vi "信号光谱9-Au-卍  -MoO3.vi"() -> ()   [LabVIEW 2018]
uses:
  <vilib>/Utility/NIReport.llb/Report Type.ctl
  <vilib>/Utility/file.llb/Write Delimited Spreadsheet (DBL).vi
  <vilib>/Instr/_visa.llb/VISA Configure Serial Port (Instr).vi
  <vilib>/addons/_office/excel.llb/Excel Get Data ([str]).vi
  <vilib>/Utility/NIReport.llb/NI_report.lvclass
  <vilib>/Analysis/NI_AALBase.lvlib
  <vilib>/ptbypt/NI_PtbyPt.lvlib
  <vilib>/Utility/NIReport.llb/NI_ReportGenerationCore.lvlib
  <vilib>/addons/_office/NI_ReportGenerationToolkit.lvlib
  <vilib>/Utility/NIReport.llb/Excel/NI_Excel.lvclass
panel:
  in  "CW":i32=1
  out "temp":i32
  in  "num":i32=2
  in  "角度判断下限":dbl=1.0 format="%#_13g"
  in  "角度判断上限":dbl=4.0 format="%#_13g"
  out "原始峰值":dbl
  out "拟合峰值":dbl
  in  "角度倍乘系数":dbl=1.5
  out "结果展示":dbl[][](array[numeric])=[[37.33100777239877, 2672.955043835526, 29.54153292599307, 222755.0, 50.0], [37.36593979472361, 2672.656498058864, 30.113284142729572, 222833.0, 50.0], [38.96986225690859, 2673.3337152325566, 33.38805102415213, 222910.0, 75.0], [37.39946104045098, 2676.4005085744548, 31.215565446104666, 222948.0, 47.0], [35.862209164247574, 2671.7826876859012, 30.355582265151796, 223028.0, 47.0]]
  out "Δw2>C":bool=TRUE
  out "Δw1>C":bool=TRUE
  out "θi":dbl
  in  "w0":dbl format="%#_13g"
  in  "C=w-w0":dbl=1800.0 format="%#_13g"
  in  "上升下降沿/s":dbl format="%.2p"
  in  "延时/s":dbl format="%.2p"
  in  "占空比/%":dbl=3.0 format="%.2p"
  in  "高电平/V":dbl=4.0 format="%.2p"
  in  "频率/Hz":dbl=6000.0 format="%.3p"
  in  "低电平/V":dbl min=0.0 max=5.0 format="%.2p"
  in  "Enable":bool
  in  "上升下降沿":i32(ring)=1 items=["上升沿", "下降沿"]
  in  "输出信号波形":u16(ring) items=["Pulse"]
  out "Output":bool
  in  "VISA 信号发生器":refnum<visa-resource-name>="USB0::0x1AB1::0x0641::DG4E192200870::INSTR"
  out "Output 2":bool
  in  "Enable 2":bool
  in  "上升下降沿/s 2":dbl format="%.2p"
  in  "延时/s 2":dbl format="%.2p"
  in  "占空比/% 2":dbl=3.0 format="%.2p"
  in  "高电平/V 2":dbl=0.002 format="%.2p"
  in  "频率/Hz 2":dbl=6000.0 format="%.3p"
  in  "低电平/V 2":dbl min=0.0 max=5.0 format="%.2p"
  in  "上升下降沿 2":i32(ring)=1 items=["上升沿", "下降沿"]
  in  "输出信号波形 2":u16(ring) items=["Pulse"]
  in  "终止测量":bool
  in  "测量次数":i32=1
  out "best fit":cluster{"Y":dbl[], "Y":dbl[]}[](graph)
  in  "拟合终点":i32=850
  in  "拟合起点":i32=200
  out "angle":dbl
  out "图片地址":string
  in  "开光时间/ms":u32=50
  out "最终存储路径 2":path
  out "照明光error out":errorcluster
  in  "照明光":bool
  in  "stop bits (10: 1 bit)":u16(ring)=10 items=["1.0"=10, "1.5"=15, "2.0"=20]
  in  "parity (0:none)":enum16{"None", "Odd", "Even", "Mark", "Space"}(ring)
  in  "data bits (8)":u16=8 min=5 max=8 step=1
  in  "baud rate":u32=9600 caption="baud rate (115200)" min=9600 max=115200
  in  "照明光VISA":refnum<visa-resource-name>="COM13"
  out "正在测量":bool
  in  "滤波阈值":dbl=3000.0 format="%#_13g"
  out "范围内？":bool[](array[boolean])
  out "w":dbl
  out "xc":dbl
  out "拟合参数":dbl[](array[numeric])
  out "最终存储路径":path
  in  "停止程序":bool
  out "configure error out":errorcluster
  in  "设置参数":bool
  out "output control error  4":errorcluster
  in  "低电平持续输出":bool
  out "output control error  5":errorcluster
  out "output control error":errorcluster
  in  "开始测量":bool
  in  "channel输出口":i32(ring) items=["Channel 1", "Channel 2"]
  out "output control error":errorcluster
  out "Spectrum":cluster{"Y":dbl[], "Y":dbl[]}[](graph)
  out "波长范围":dbl[](array[numeric])
  in  "?":enum32{"IHR 550", "CCD"}(tab)
  in  "Move To\nTarget Positions":bool
  out "Current UniqueID":string="Mono4"
  in  "Mono ID":string(combo)="Mono1"
  in  "Connect":bool
  out "Initialized JY":bool=TRUE
  in  "Force\nInitialization":bool
  in  "Target Grating":string(combo)="2"
  out "Current Description":string="1" caption="Description"
  out "Grating Index":i32=1
  out "Current Grating":dbl=1200.0
  out "Units":string="nm"
  out "Current WL":dbl=897.9988
  out "Exit Mirror\nPosition":i32(ring)=2 items=["EntranceMirror", "ExitMirror", "Front", "Side"]
  out "Entrance Mirror\nPosition":i32(ring)=2 items=["EntranceMirror", "ExitMirror", "Front", "Side"]
  out "Units 2":string="mm"
  out "Front Entrance":dbl
  in  "Target WL":dbl=516.0
  in  "Exit Mirror":u16(ring)=3 caption="Target Position Exit Mirror" items=["Front"=2, "Side"=3]
  in  "Entrance Mirror":u16(ring)=2 caption="Target Position\nEntrance Mirror" items=["Front"=2, "Side"=3]
  in  "Target\nFront Entrance":dbl=2.0
  in  "Commande tab":T1(tab)
  in  "Area Number to Display":i32
  in  "Reformat":bool
  in  "GAIN":u16(ring)=2 caption="Device Name" items=["High Light", "Best Dynamic Range", "High Sensitivity"]
  in  "ADC":u16(ring) caption="Device Name" items=["20 kHz       ", " 1 MHz       ", " 1 MHz Ultra "]
  in  "Number of Areas :":u16=1 min=1 step=1
  in  "Integration time (ms) :":i16=5000
  out "Uniques ID":u16(ring) items=["CCD1", "CCD2"]
  in  "Device Name":u16(ring) items=["Synapse CCD (Lateral)", "Synapse_IGA (Axial)"]
  in  "Signal type :":enum16{"TTL Rising Edge", "TTL Falling Edge"}(ring)=enum."TTL Falling Edge"
  in  "Trigger Type :":u16(ring) items=["On Start"=1, "Per Acquisition"=2]
  in  "trigSigTypeString":string
  in  "trigEventString":string
  in  "Enable InputTriggers :":bool
  in  "Number of Cleans":i32=1
  in  "MultiAcqShutterMode":i32(ring)=3 items=["Open For All Spectra"=1, "Open for Each Spectrum"=3]
  in  "Accumulations:":u16=10 min=1 step=1
  in  "Multi Accumulation mode:":bool
  out "Y Pixels:":i32=256
  out "DataSize":i32=1024
  out "X Pixels:":i32=1024
  out "Firmware\nVersion":string="V1.20 CCD_4000"
  out "initialized ?":bool=TRUE
  in  "Continuous":bool
  in  "CCD Busy":bool
  out "indicator":string="Ready !"
  in  "initialize":bool
  in  "ShutterOpen":bool=TRUE caption="Shutter enable"
  in  "Acquire":bool
  in  "Temperature":bool
  in  "Setup":bool
  out "Acq Time(ms)":u32=3401
  in  "Save Backlight":bool
  in  "cut backlight":bool
  out "backlight":bool=TRUE
  in  "是否拟合":bool
  in  "是否保存":bool
  in  "Close":bool=TRUE
  out "JYCCDLib.IJYCCDReqd":refnum<k7>
  out "areas :":i32[][](array[numeric])=[[1], [1], [1], [1024], [256], [1], [256]]
  in  "Constante de condition\n(Voir l'aide contextuelle)":bool
  out "temp graph":dbl(graph)=-134.538067
  out "ADC Number":i32[](array[numeric])=[0, 1, 2, 3, 4]
  out "Gain Number":i32[](array[numeric])=[10, 11, 12, 13, 8, 2]
  out "trigAddress":i32
  out "Data":i32[][](graph)
  out "error out":errorcluster
  out "Gratings":dbl[](array[numeric])=[1200.0, 300.0]
  out "Backlight":i32[][](graph)
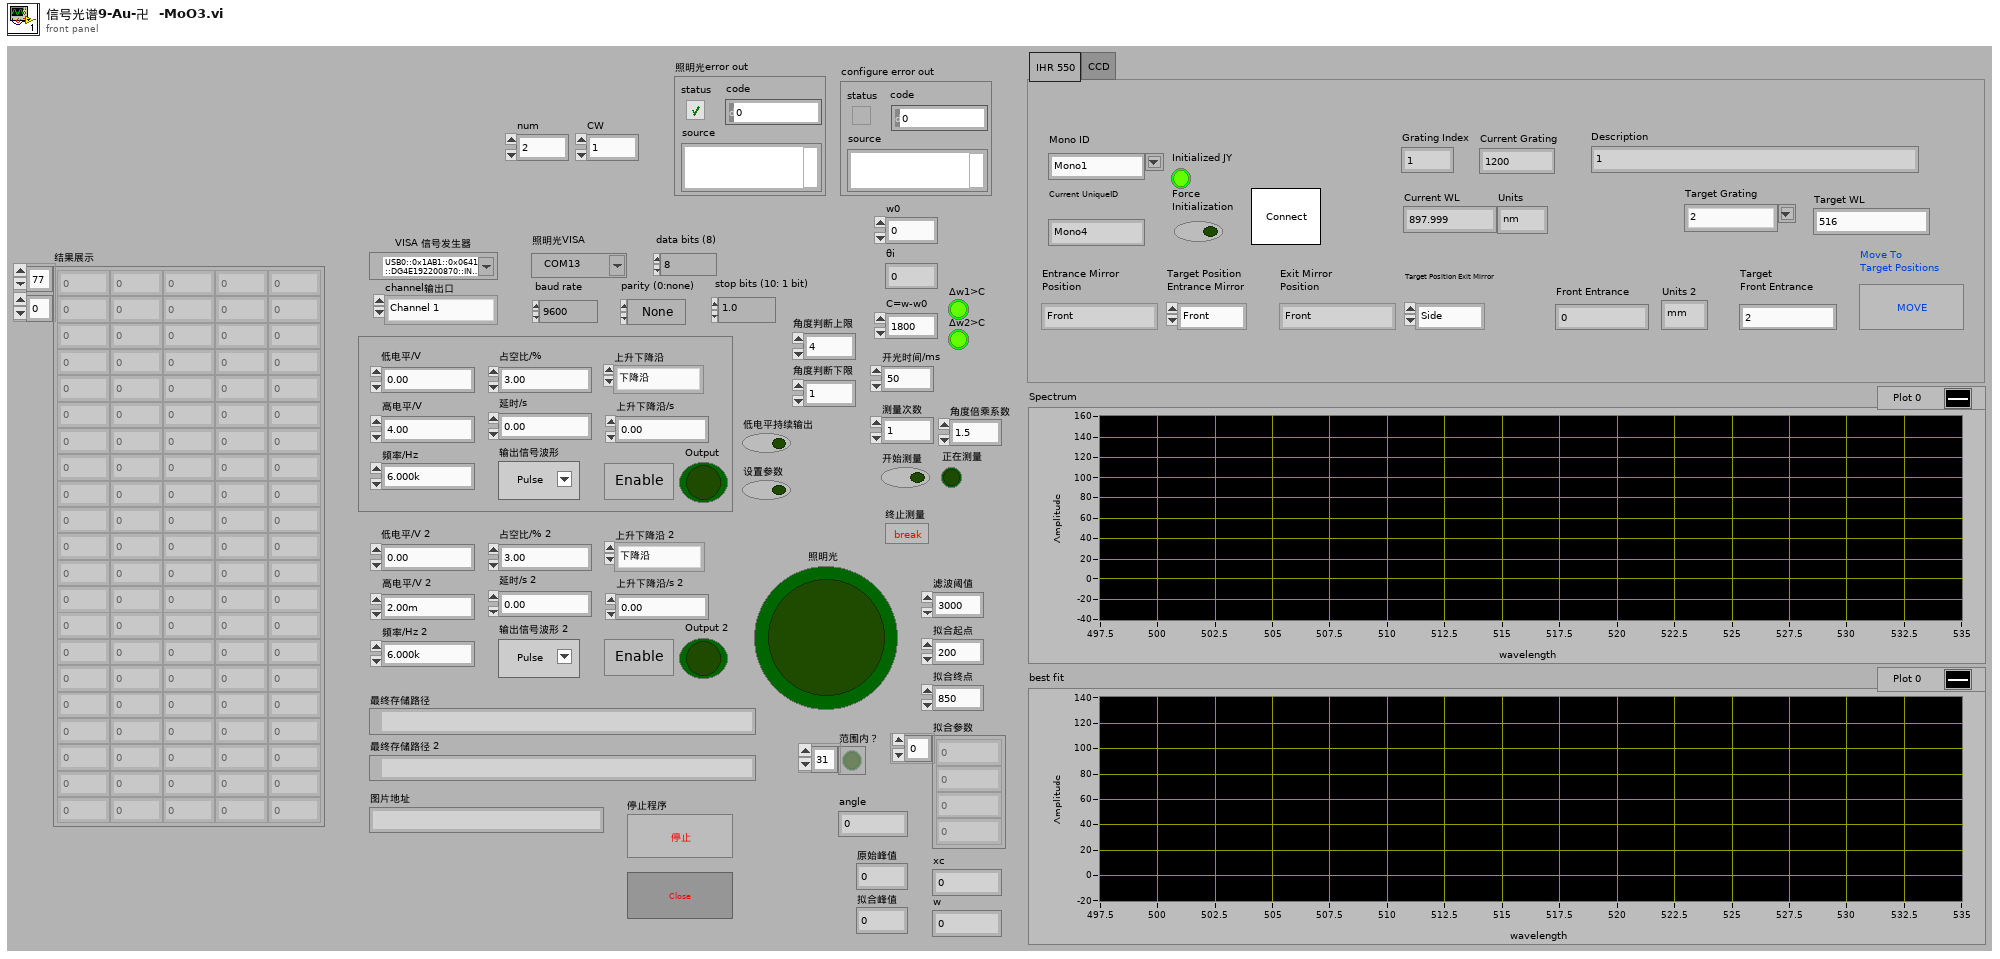
[diagram p1: front panel]
types:
  T1 = enum32{"Settings", "Trigger In", "Multi-Accu.", "Infos"}
  T2 = enum8{"Enabled", "Disabled", "Disabled and Grayed Out"}
  T3 = enum16{"maximized", "minimized", "normal", "no change"}
  T4 = typedef "NI_ReportGenerationCore.lvlib/Report Type.ctl" = enum16{"HTML", "Word", "Excel"}
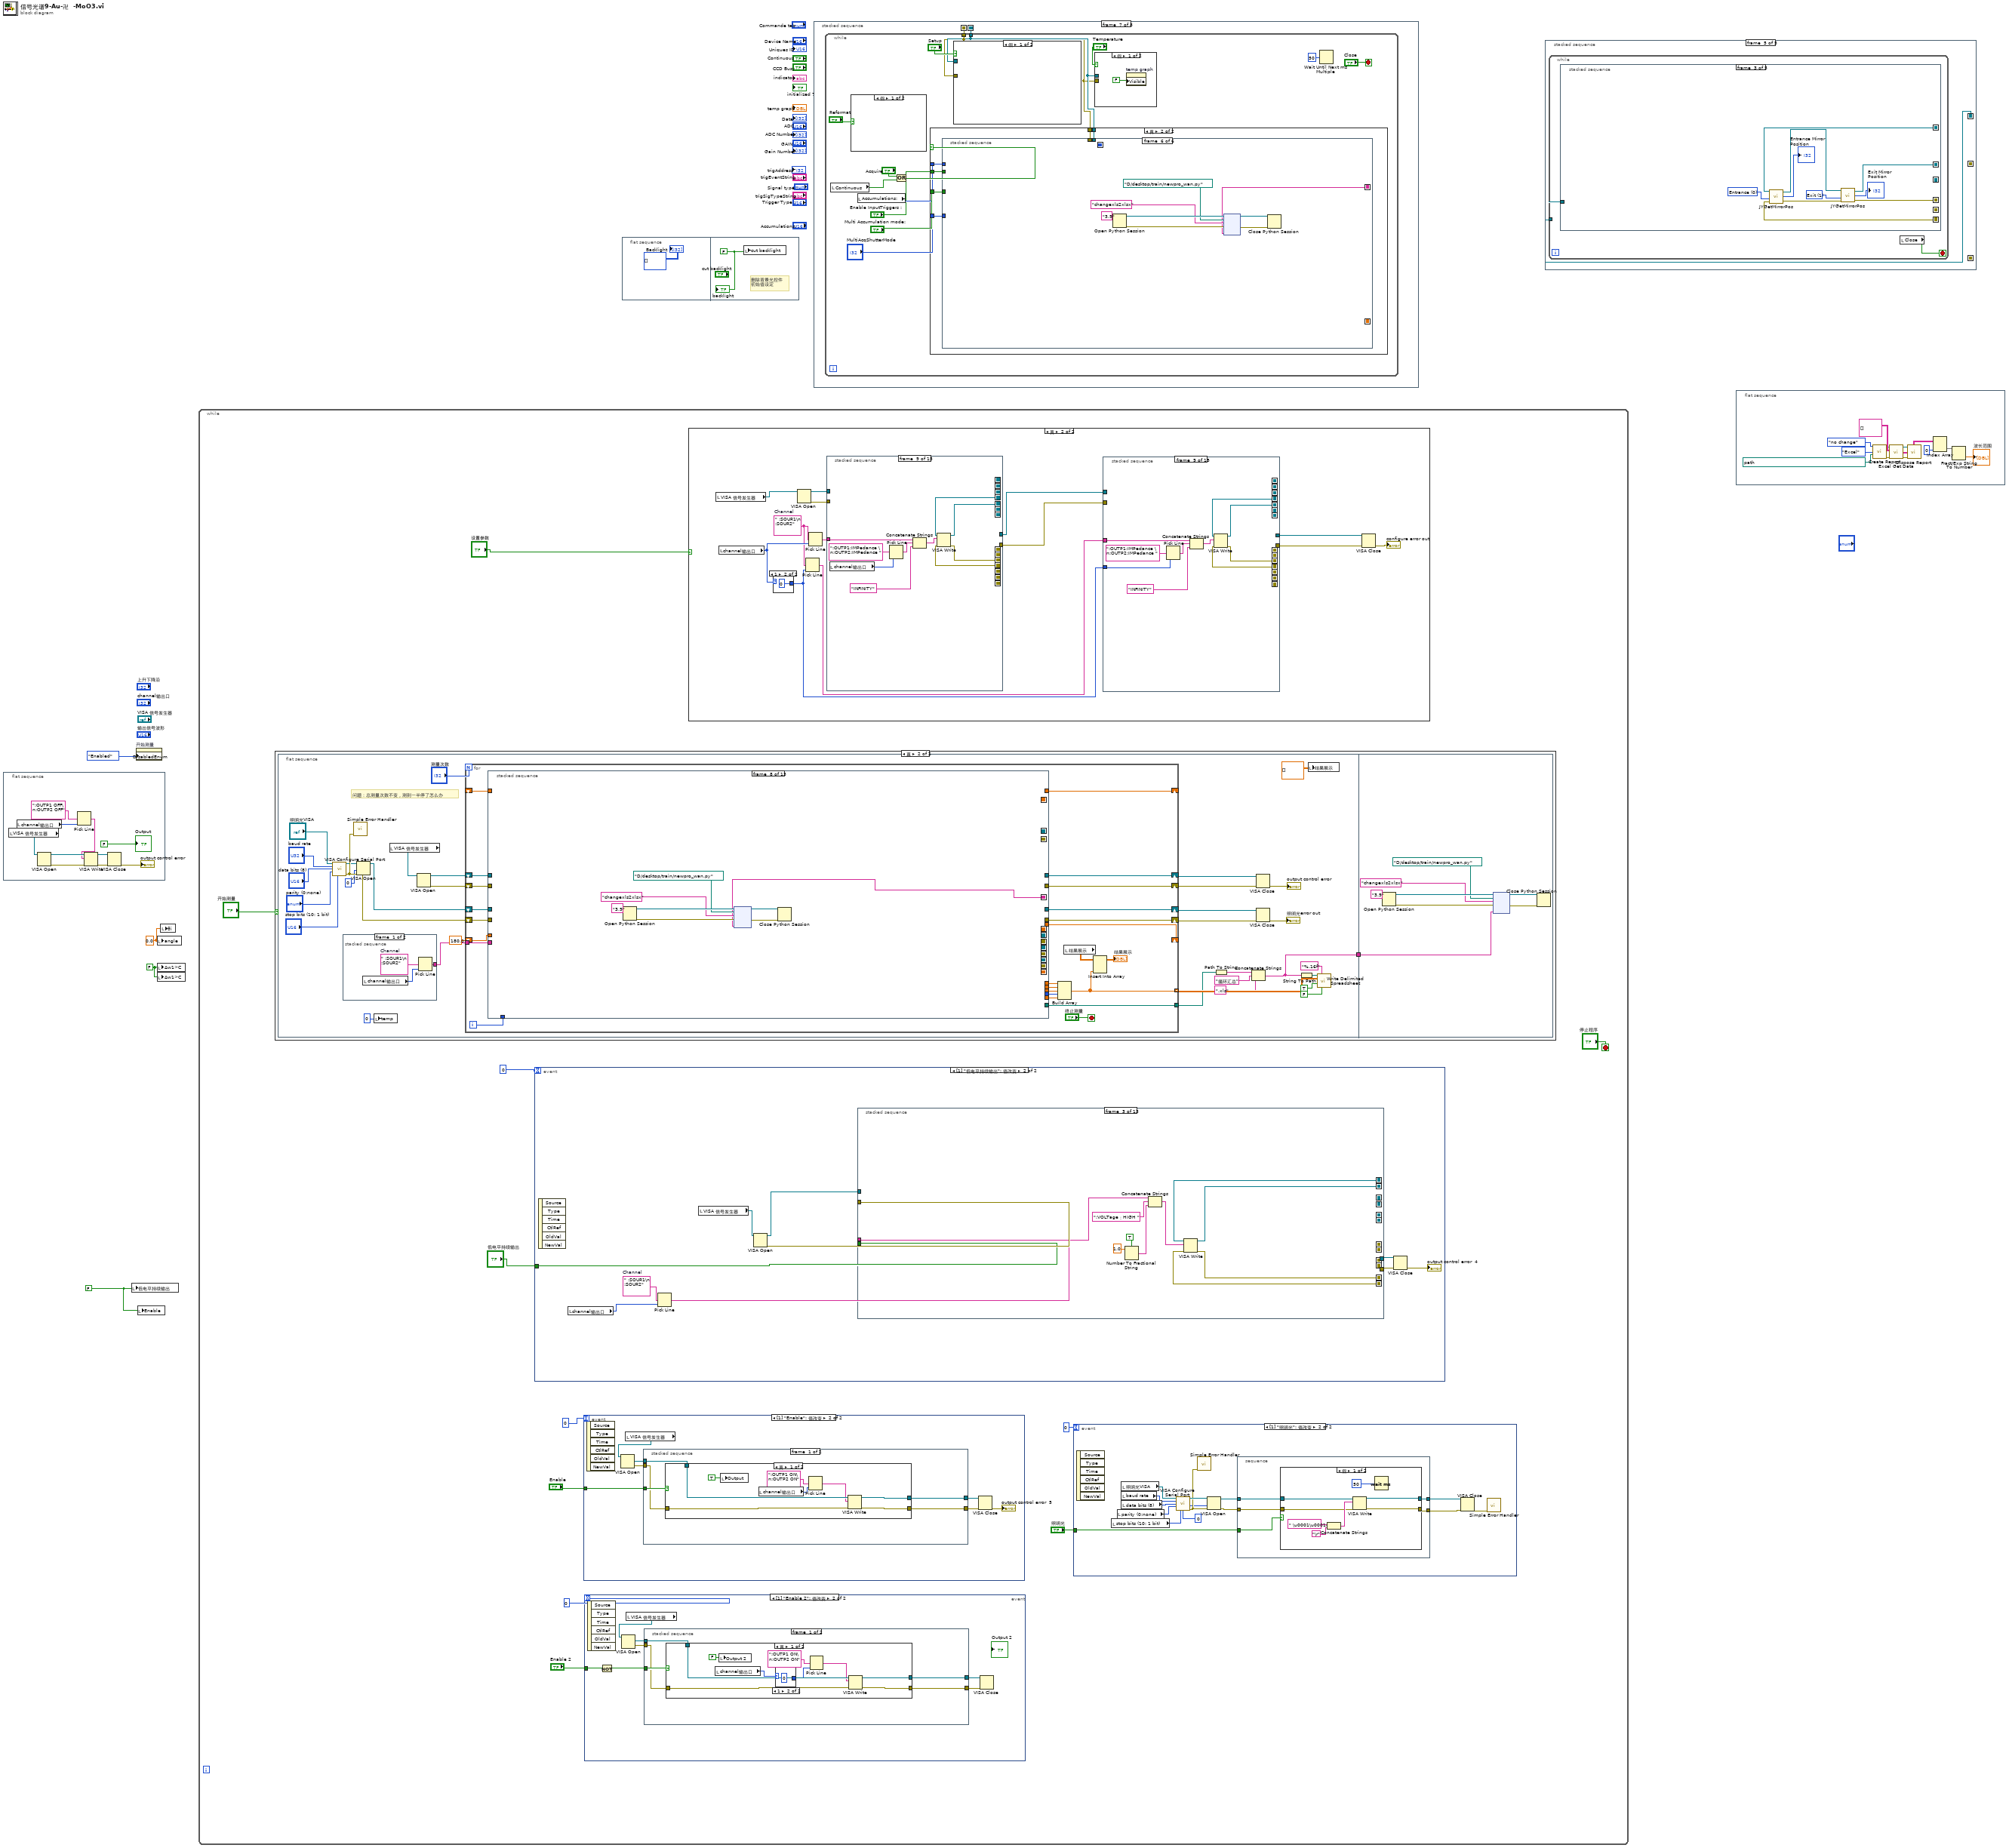
[diagram p0: block diagram]
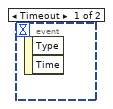
[diagram p2: hidden frame]
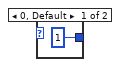
[diagram p3: hidden frame]
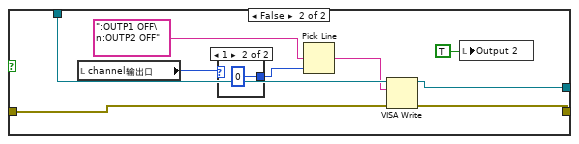
[diagram p4: hidden frame]
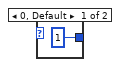
[diagram p5: hidden frame]
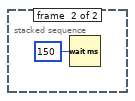
[diagram p6: hidden frame]
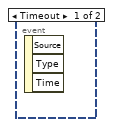
[diagram p7: hidden frame]
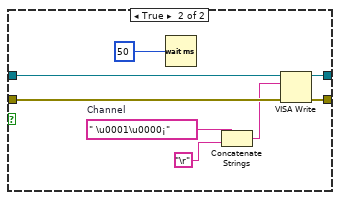
[diagram p8: hidden frame]
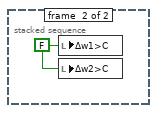
[diagram p10: hidden frame]
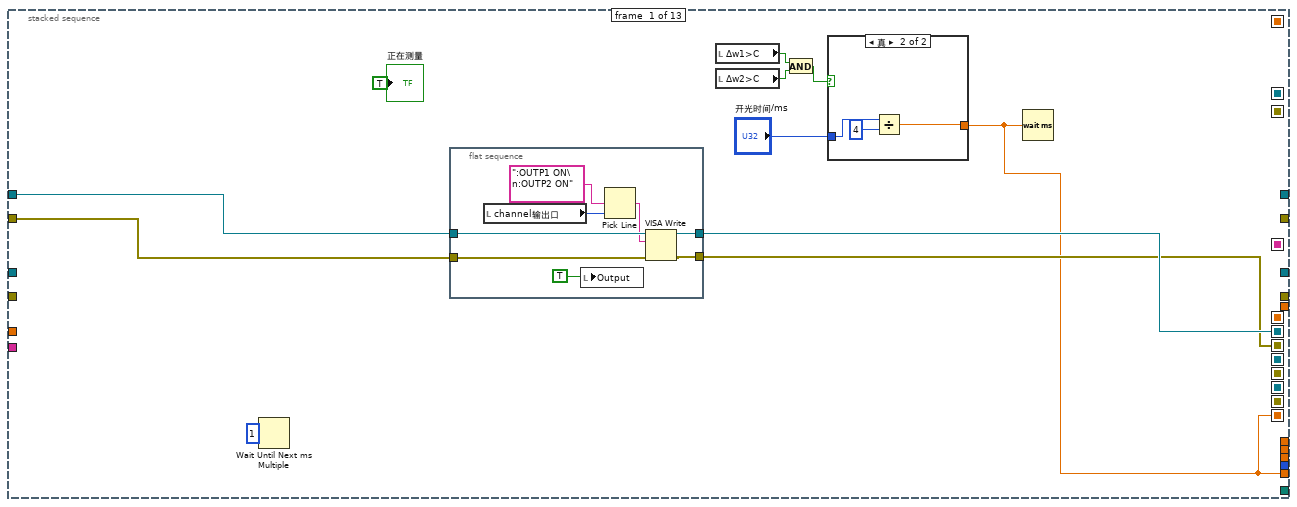
[diagram p11: hidden frame]
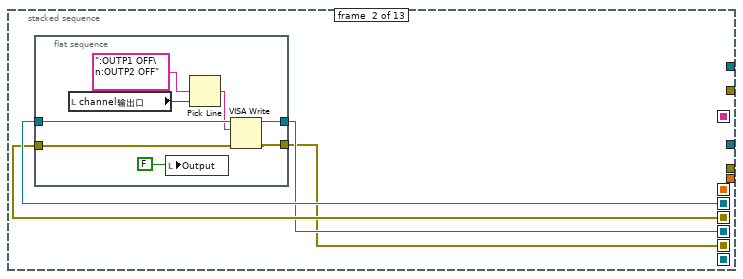
[diagram p13: hidden frame]
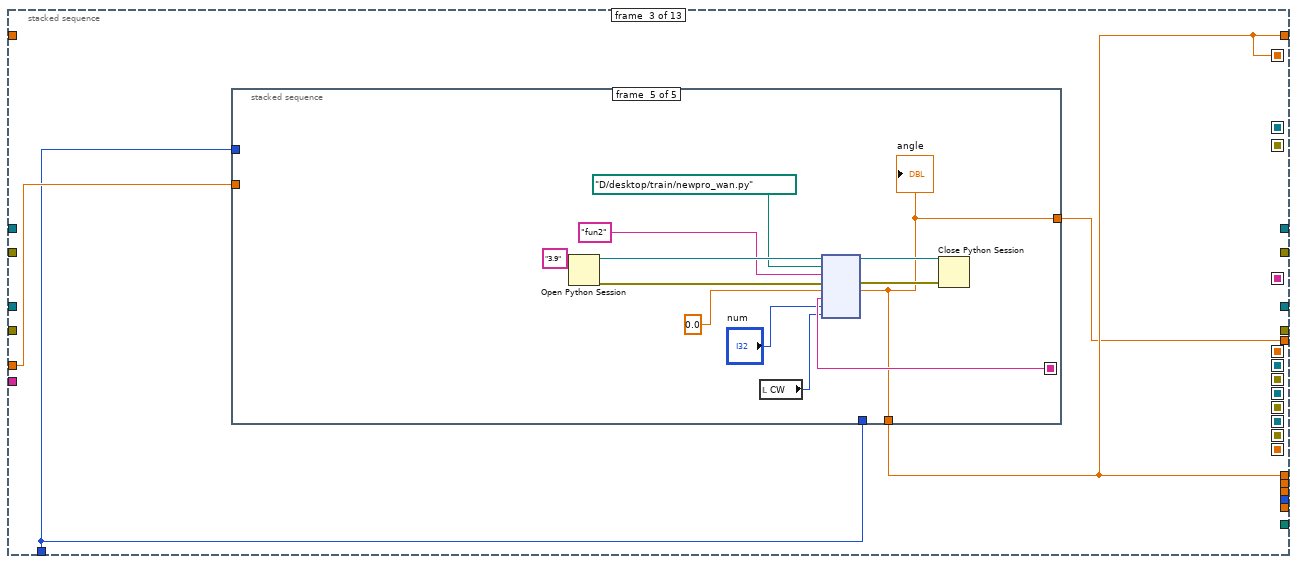
[diagram p14: hidden frame]
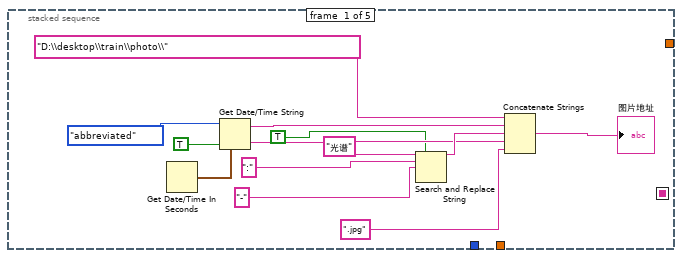
[diagram p15: hidden frame]
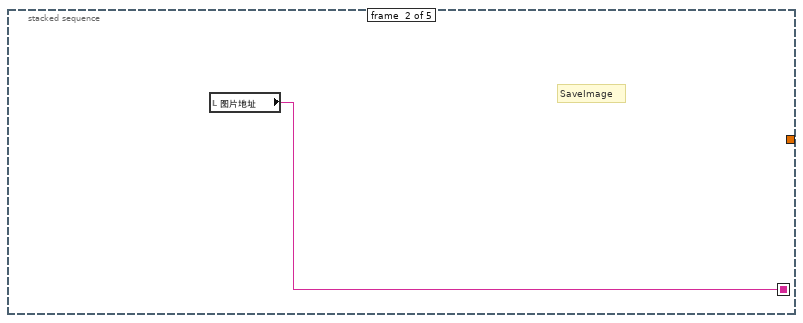
[diagram p16: hidden frame]
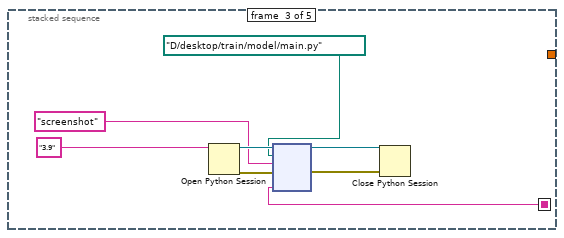
[diagram p17: hidden frame]
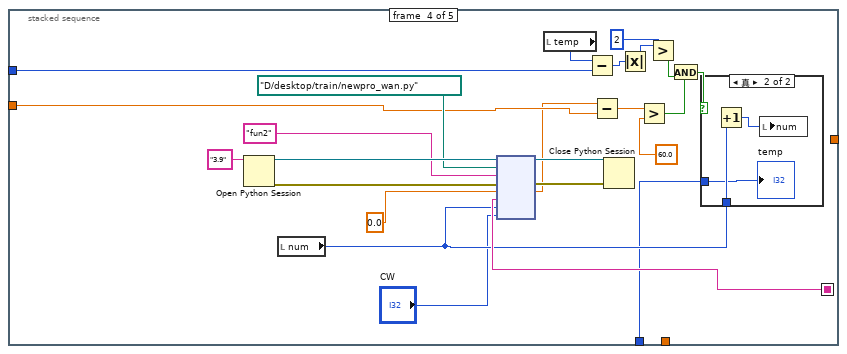
[diagram p18: hidden frame]
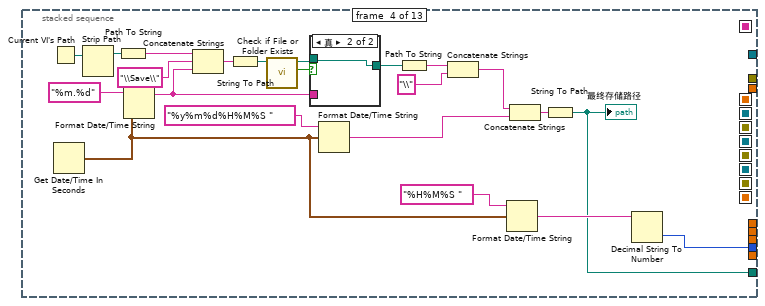
[diagram p20: hidden frame]
diagram:
  w1 = FALSE ("Δw1>C")
  w2 = 0.0 ("angle")
  w3 = FALSE
  n1 = flat-sequence {
    frame #0 {
      n2 = local read "VISA 信号发生器"() -> (w8:refnum<visa-resource-name>)
      n3 = local read "channel输出口"() -> (w6:i32)
      n4 = VISA Open(VISA resource name=w8) -> (VISA resource name=w14:refnum<visa-resource-name>, error out=w13:errorcluster)  [unwired: 4 in]
      n5 = Pick Line(multi-line string=":OUTP1 OFF\n:OUTP2 OFF" ("write buffer"), line index=w6) -> (output string=w5:string)  [unwired: 1 in]
      n6 = VISA Write(VISA resource name=w14, write buffer=w5, error in (no error)=w13) -> (VISA resource name out=w11:refnum<visa-resource-name>, error out=w10:errorcluster)  [unwired: 1 out]
      n7 = VISA Close(VISA resource name=w11, error in (no error)=w10) -> (error out=→"output control error":errorcluster)
      "Output" <- FALSE ("布尔")
    }
  }
  n8 = local write "低电平持续输出"(w3) -> ()
  n9 = property on="开始测量" class="Bool"("DisabledEnum"=T2."Enabled" ("禁用")) -> ()  [unwired: 2 in, 2 out]
  n10 = local write "Enable"(w3) -> ()
  n11 = local write "angle"(w2) -> ()
  n12 = local write "Δw1>C"(w1) -> ()
  n13 = local write "Δw1>C"(w1) -> ()
  n14 = local write "θi"(w2) -> ()
  n15 = while {
    stop <- "停止程序" stop-if-true
    n16 = case shown="真" "开始测量" {
      frame False {
      }
      frame True {
        n17 = flat-sequence {
          tunnel: [w97] -> w96
          tunnel: w96 -> [w500]
          frame #0 {
            # "问题：总测量次数不变，测到一半停了怎么办"
            n18 = call-poly "VISA Configure Serial Port"("VISA resource name"="照明光VISA", "baud rate (9600)"="baud rate", "data bits (8)"="data bits (8)", "parity (0:none)"="parity (0:none)", "stop bits (10: 1 bit)"="stop bits (10: 1 bit)") -> ("VISA resource name out"=w121:refnum<visa-resource-name>, "error out"=w122:errorcluster)  [unwired: 9 in]
            n19 = stacked-sequence {
              tunnel: [w131 _] -> w125
              frame #0 {
                w132 = " :SOUR1\n :SOUR2"  # Channel
                n20 = local read "channel输出口"() -> (w133:i32)
                n21 = Pick Line(multi-line string=w132, line index=w133) -> (output string=w131:string)  [unwired: 1 in]
              }
              frame #1 {
                w134 = FALSE ("Δw1>C")
                n22 = local write "Δw1>C"(w134) -> ()
                n23 = local write "Δw2>C"(w134) -> ()
              }
            }
            n24 = call <vilib>:"Simple Error Handler.vi"("error in (no error)"=w122) -> ()  [unwired: 4 in, 5 out]
            n25 = VISA Open(access mode=0, error in (no error)=w122, VISA resource name=w121) -> (VISA resource name=w114:refnum<visa-resource-name>, error out=w113:errorcluster)  [unwired: 2 in]
            n26 = local write "temp"(0 ("temp")) -> ()
            n27 = local read "VISA 信号发生器"() -> (w130:refnum<visa-resource-name>)
            n28 = VISA Open(VISA resource name=w130) -> (VISA resource name=w129:refnum<visa-resource-name>, error out=w128:errorcluster)  [unwired: 4 in]
            n29 = for {
              N: "测量次数" -> [_]
              tunnel: w125 -> [w156]
              shift-right: [w152] -> w124
              shift-left: w129 -> [w158]
              shift-right: [w151] -> w123
              shift-left: w128 -> [w157]
              shift-right: [w150] -> w127
              shift-left: w114 -> [w155]
              shift-right: [w149] -> w126
              shift-left: w113 -> [w154]
              tunnel: [w139] -> w104 mode=indexing
              shift-right: [w144] -> _
              shift-left: _ -> [w143]
              tunnel: [w140] -> w101
              shift-right: [w136] -> _
              shift-left: 180.0 -> [w135]
              i -> [w142]
              stop <- "终止测量" stop-if-true
              n30 = stacked-sequence {
                seq-local: [w165 _ _ _ _ _ _ _ _ _ _ _ _] -> [_ w185 _ _ _ _ _ _ _ _ _ _ _]
                seq-local: [w164 _ _ _ _ _ _ _ _ _ _ _ _] -> [_ w184 _ _ _ _ _ _ _ _ _ _ _]
                seq-local: [_ _ _ _ _ w302 _ _ _ _ _ _ _] -> [_ _ _ _ _ _ _ _ _ w428 _ _ _]
                seq-local: [_ _ _ _ _ w301 _ _ _ _ _ _ _] -> [_ _ _ _ _ _ _ _ _ w431 _ _ _]
                seq-local: [_ w183 _ _ _ _ _ _ _ _ _ _ _] -> [_ _ _ _ w288 _ _ _ _ _ _ _ _]
                seq-local: [_ w182 _ _ _ _ _ _ _ _ _ _ _] -> [_ _ _ _ w287 _ _ _ _ _ _ _ _]
                seq-local: [_ _ _ _ w286 _ _ _ _ _ _ _ _] -> [_ _ _ _ _ _ _ _ w414 _ _ _ _]
                seq-local: [_ _ _ _ w285 _ _ _ _ _ _ _ _] -> [_ _ _ _ _ _ _ _ w413 _ _ _ _]
                seq-local: [_ _ w197 _ _ _ _ _ _ _ _ _ _] -> [_ _ _ _ _ _ _ _ _ _ _ w440 _]
                seq-local: [_ _ _ _ _ _ w316 _ _ _ _ _ _] -> [_ _ _ _ _ _ _ _ _ _ _ w435 _]
                seq-local: [w159 _ _ _ _ _ _ _ _ _ _ _ _] -> [_ _ _ _ _ _ w314 _ _ _ _ _ _]
                seq-local: [_ _ _ _ _ _ w309 _ _ _ _ _ _] -> [_ _ _ _ _ _ _ w403 _ _ _ _ _]
                tunnel: w158 -> [w167 _ _ _ _ _ _ _ _ _ _ _ _]
                tunnel: w157 -> [w166 _ _ _ _ _ _ _ _ _ _ _ _]
                tunnel: [_ _ _ _ _ _ _ _ w412 _ _ _ _] -> w152
                tunnel: [_ _ _ _ _ _ _ _ w411 _ _ _ _] -> w151
                tunnel: w156 -> [_ _ _ _ _ _ _ _ _ _ _ _ _]
                tunnel: w155 -> [_ _ _ _ _ w305 _ _ _ _ _ _ _]
                tunnel: w154 -> [_ _ _ _ _ w304 _ _ _ _ _ _ _]
                tunnel: [_ _ _ _ _ _ _ _ _ w430 _ _ _] -> w150
                tunnel: [_ _ _ _ _ _ _ _ _ w429 _ _ _] -> w149
                tunnel: [_ _ w197 _ _ _ _ _ _ _ _ _ _] -> w148
                tunnel: [_ _ _ _ _ _ w311 _ _ _ _ _ _] -> w147
                tunnel: [_ _ _ _ _ _ w310 _ _ _ _ _ _] -> w146
                tunnel: [_ _ _ w260 _ _ _ _ _ _ _ _ _] -> w145
                tunnel: [w159 _ _ _ _ _ _ _ _ _ _ _ _] -> w141
                tunnel: [_ _ w197 _ _ _ _ _ _ _ _ _ _] -> w144
                tunnel: w143 -> [_ _ _ _ _ _ _ _ _ _ _ w439 _]
                tunnel: w142 -> [_ _ w194 _ _ _ _ _ _ _ _ w437 _]
                tunnel: [_ _ _ w259 _ _ _ _ _ _ _ _ _] -> w140
                tunnel: [_ _ w196 _ _ _ _ _ _ _ _ _ _] -> w136
                tunnel: w135 -> [_ _ w195 _ _ _ _ _ _ _ _ _ _]
                frame #0 {
                  n31 = Wait Until Next ms Multiple(millisecond multiple=u32 1 ("毫秒倍数")) -> ()  [unwired: 1 out]
                  n32 = flat-sequence {
                    tunnel: w167 -> [w181]
                    tunnel: w166 -> [w180]
                    tunnel: [w175] -> w165
                    tunnel: [w174] -> w164
                    frame #0 {
                      n33 = local read "channel输出口"() -> (w177:i32)
                      n34 = local write "Output"(TRUE ("布尔")) -> ()
                      n35 = Pick Line(multi-line string=":OUTP1 ON\n:OUTP2 ON" ("write buffer"), line index=w177) -> (output string=w176:string)  [unwired: 1 in]
                      n36 = VISA Write(VISA resource name=w181, write buffer=w176, error in (no error)=w180) -> (VISA resource name out=w175:refnum<visa-resource-name>, error out=w174:errorcluster)  [unwired: 1 out]
                    }
                  }
                  n37 = local read "Δw1>C"() -> (w161:bool)
                  n38 = local read "Δw2>C"() -> (w162:bool)
                  n39 = And(x=w161, y=w162) -> (x .and. y?=w160:bool)
                  n40 = case shown="真" w160 {
                    tunnel: [w170 w171] -> w159
                    tunnel: "开光时间/ms" -> [w170 w173]
                    frame False {
                    }
                    frame True {
                      n41 = Divide(x=w173, y=u32 4) -> (x/y=w171:dbl)
                    }
                  }
                  n42 = Wait (ms)(milliseconds to wait=w159) -> ()  [unwired: 1 out]
                  "正在测量" <- TRUE
                }
                frame #1 {
                  n43 = flat-sequence {
                    tunnel: w185 -> [w193]
                    tunnel: w184 -> [w192]
                    tunnel: [w187] -> w183
                    tunnel: [w186] -> w182
                    frame #0 {
                      n44 = local read "channel输出口"() -> (w189:i32)
                      n45 = local write "Output"(FALSE ("布尔")) -> ()
                      n46 = Pick Line(multi-line string=":OUTP1 OFF\n:OUTP2 OFF" ("write buffer"), line index=w189) -> (output string=w188:string)  [unwired: 1 in]
                      n47 = VISA Write(VISA resource name=w193, write buffer=w188, error in (no error)=w192) -> (VISA resource name out=w187:refnum<visa-resource-name>, error out=w186:errorcluster)  [unwired: 1 out]
                    }
                  }
                }
                frame #2 {
                  n48 = stacked-sequence {
                    seq-local: [_ w211 _ _ _] -> [_ _ w212 w235 w250]
                    tunnel: [_ _ _ _ w248] -> w197
                    tunnel: [_ _ _ _ w248] -> w196
                    tunnel: w195 -> [_ _ _ w231 _]
                    tunnel: w194 -> [_ _ _ w227 _]
                    tunnel: w194 -> [_ _ _ w225 _]
                    frame #0 {
                      n49 = Get Date/Time In Seconds() -> (seconds since 1Jan1904=w207:timestamp)
                      n50 = Get Date/Time String(date format (0)=enum16{"short", "long", "abbreviated"}."abbreviated" ("日期格式(0)"), seconds (now)=w207, want seconds? (F)=TRUE ("需要秒？(F)")) -> (date string=w210:string, time string=w208:string)
                      n51 = Search and Replace String(replace all?=TRUE ("替换全部？(F)"), input string=w208, search string=":" ("搜索字符串"), replace string="-" ("替换字符串(\"\")")) -> (result string=w209:string)  [unwired: 4 in, 3 out]
                      n52 = Concatenate Strings("D:\\desktop\\train\\photo\\", w210, w209, "光谱" ("字符串"), ".jpg" ("字符串")) -> (→"图片地址":string)
                    }
                    frame #1 {
                      # "SaveImage"
                      n53 = local read "图片地址"() -> (w211:string)
                    }
                    frame #2 {
                      n54 = Open Python Session(python version="3.9" ("Python version")) -> (session out=w219:refnum<k35>, error out=w217:errorcluster)  [unwired: 2 in]
                      n55 = node(w219, path "D:/desktop/train/model/main.py" ("module path"), "screenshot" ("function name"), w217, w212) -> (w218:refnum<k35>, w216:errorcluster)  [unwired: 3 in, 2 out]
                      n56 = Close Python Session(session in=w218, error in=w216) -> ()  [unwired: 1 out]
                    }
                    frame #3 {
                      n57 = Open Python Session(python version="3.9" ("Python version")) -> (session out=w242:refnum<k35>, error out=w240:errorcluster)  [unwired: 2 in]
                      n58 = local read "num"() -> (w232:i32)
                      n59 = node(w242, path "D:/desktop/train/newpro_wan.py" ("module path"), "fun2" ("function name"), w240, 0.0, w235, w232, "CW") -> (w241:refnum<k35>, w239:errorcluster, w230:dbl)  [unwired: 3 in, 2 out]
                      n60 = local read "temp"() -> (w226:i32)
                      n61 = Subtract(x=w226, y=w225) -> (x-y=w224:i32)
                      n62 = Subtract(x=w230, y=w231) -> (x-y=w234:dbl)
                      n63 = Close Python Session(session in=w241, error in=w239) -> ()  [unwired: 1 out]
                      n64 = Absolute Value(x=w224) -> (abs(x)=w223:i32)
                      n65 = Greater?(x=w234, y=60.0) -> (0:w229:bool)
                      n66 = Greater?(x=w223, y=2) -> (0:w222:bool)
                      n67 = And(x=w229, y=w222) -> (x .and. y?=w228:bool)
                      n68 = case shown="真" w228 {
                        tunnel: w232 -> [_ w246]
                        tunnel: w227 -> [_ w244]
                        frame False {
                        }
                        frame True {
                          n69 = Increment(x=w246) -> (x+1=w245:i32)
                          n70 = local write "num"(w245) -> ()
                          "temp" <- w244
                        }
                      }
                    }
                    frame #4 {
                      n71 = Open Python Session(python version="3.9" ("Python version")) -> (session out=w257:refnum<k35>, error out=w255:errorcluster)  [unwired: 2 in]
                      n72 = local read "CW"() -> (w247:i32)
                      n73 = node(w257, path "D:/desktop/train/newpro_wan.py" ("module path"), "fun2" ("function name"), w255, 0.0, w250, "num", w247) -> (w256:refnum<k35>, w254:errorcluster, w248:dbl)  [unwired: 3 in, 2 out]
                      "angle" <- w248
                      n74 = Close Python Session(session in=w256, error in=w254) -> ()  [unwired: 1 out]
                    }
                  }
                }
                frame #3 {
                  n75 = Current VI's Path() -> (path=w269:path)
                  n76 = Get Date/Time In Seconds() -> (seconds since 1Jan1904=w262:timestamp)
                  n77 = Strip Path(path=w269) -> (stripped path=w270:path)  [unwired: 1 out]
                  n78 = Path To String(path=w270) -> (string=w271:string)
                  n79 = Format Date/Time String(time format string (%c)="%m.%d" ("时间格式字符串(%c)"), seconds (now)=w262) -> (date/time string=w277:string)  [unwired: 1 in]
                  n80 = Concatenate Strings(w271, "\\Save\\" ("字符串"), w277) -> (w272:string)
                  n81 = String To Path(string=w272) -> (path=w273:path)
                  n82 = call <vilib>:"Check if File or Folder Exists.vi"("path"=w273) -> ("file or folder exists?"=w274:bool, "dup path"=w276:path)  [unwired: 8 in, 1 out]
                  n83 = case shown="真" w274 {
                    tunnel: [w283 w284] -> w275
                    tunnel: w276 -> [w282 w284]
                    tunnel: w277 -> [w281 _]
                    frame False {
                      n84 = Create Folder(prompt (Create Folder)=w281, path (use dialog)=w282) -> (created path=w283:path)  [unwired: 1 in, 2 out]
                    }
                    frame True {
                    }
                  }
                  n85 = Format Date/Time String(time format string (%c)="%y%m%d%H%M%S " ("时间格式字符串(%c)"), seconds (now)=w262) -> (date/time string=w280:string)  [unwired: 1 in]
                  n86 = Path To String(path=w275) -> (string=w278:string)
                  n87 = Concatenate Strings(w278, "\\" ("字符串")) -> (w279:string)
                  n88 = Format Date/Time String(time format string (%c)="%H%M%S " ("时间格式字符串(%c)"), seconds (now)=w262) -> (date/time string=w261:string)  [unwired: 1 in]
                  n89 = Concatenate Strings(w279, w280) -> (w268:string)
                  n90 = String To Path(string=w268) -> (path=w259:path)
                  "最终存储路径" <- w259
                  n91 = Decimal String To Number(string=w261) -> (number=w260:i32)  [unwired: 2 in, 1 out]
                }
                frame #4 {
                  n92 = flat-sequence {
                    tunnel: w288 -> [w297]
                    tunnel: w287 -> [w296]
                    tunnel: [w292] -> w286
                    tunnel: [w291] -> w285
                    frame #0 {
                      n93 = local read "channel输出口"() -> (w290:i32)
                      n94 = case shown="1" w290 {
                        tunnel: [1 0] -> w289
                        frame 0, Default {
                        }
                        frame 1 {
                        }
                      }
                      n95 = local write "Output 2"(FALSE ("布尔")) -> ()
                      n96 = Pick Line(multi-line string=":OUTP1 OFF\n:OUTP2 OFF" ("write buffer"), line index=w289) -> (output string=w293:string)  [unwired: 1 in]
                      n97 = VISA Write(VISA resource name=w297, write buffer=w293, error in (no error)=w296) -> (VISA resource name out=w292:refnum<visa-resource-name>, error out=w291:errorcluster)  [unwired: 1 out]
                    }
                  }
                }
                frame #5 {
                  w300 = " \u0001\u0001¢"  # Channel
                  n98 = Wait (ms)(milliseconds to wait=1200) -> ()  [unwired: 1 out]
                  n99 = Concatenate Strings(w300, "\r") -> (w306:string)
                  n100 = local write "照明光"(FALSE ("照明光")) -> ()
                  n101 = VISA Write(VISA resource name=w305, write buffer=w306, error in (no error)=w304) -> (VISA resource name out=w302:refnum<visa-resource-name>, error out=w301:errorcluster)  [unwired: 1 out]
                }
                frame #6 {
                  n102 = local read "Area Number to Display"() -> (w357:i32)
                  n103 = local read "JYCCDLib.IJYCCDReqd"() -> (w353:refnum<k7>)
                  n104 = Get Date/Time In Seconds() -> (seconds since 1Jan1904=w366:timestamp)
                  n105 = local read "最终存储路径"() -> (w379:path)
                  n106 = Get Date/Time String(date format (0)=enum16{"short", "long", "abbreviated"}."abbreviated" ("日期格式(0)"), seconds (now)=w366, want seconds? (F)=TRUE ("需要秒？(F)")) -> (date string=w374:string, time string=w369:string)
                  n107 = call "MultiAccu - Acquire spectral.vi"("error in"=errorcluster {"status"=FALSE, "code"=0, "source"=""}, "Accumulations:"=u16 1, "ShutterOpen"=TRUE, "JYCCDLib.IJYCCDReqd"=w353) -> ("Acq Time(ms)"=w359:u32, "Array Out"=w358:i32[][][])  [unwired: 1 out]
                  n108 = local write "Acq Time(ms)"(w359) -> ()
                  n109 = local read "cut backlight"() -> (w341:bool)
                  n110 = local read "backlight"() -> (w339:bool)
                  n111 = Search and Replace String(replace all?=TRUE ("替换全部？(F)"), input string=w369, search string=":" ("搜索字符串"), replace string="-" ("替换字符串(\"\")")) -> (result string=w373:string)  [unwired: 4 in, 3 out]
                  n112 = Path To String(path=w379) -> (string=w363:string)
                  n113 = And(x=w341, y=w339) -> (x .and. y?=w340:bool)
                  n114 = call "Array reset dimension.vi"("Area Number"=w357, "Array In"=w358) -> ("Array Out"=w343:i32[][])
                  n115 = Concatenate Strings(w363, w374, w373, "光谱" ("字符串"), ".xls" ("字符串")) -> (w309:string)
                  n116 = case shown="真" w340 {
                    tunnel: [w399 w401] -> w342
                    tunnel: w343 -> [w399 w400]
                    frame False {
                    }
                    frame True {
                      n117 = local read "Backlight"() -> (w402:i32[][])
                      n118 = Subtract(x=w400, y=w402) -> (x-y=w401:i32[][])
                    }
                  }
                  n119 = local write "Data"(w343) -> ()
                  n120 = String To Path(string=w309) -> (path=w378:path)
                  n121 = local read "波长范围"() -> (w322:dbl[])
                  n122 = Index Array(array=w342, index (row)=0 ("索引 (行)")) -> (element=w380:i32[])  [unwired: 1 in]
                  n123 = Reverse 1D Array(array=w380) -> (reversed array=w319:i32[])
                  n124 = local read "angle"() -> (w321:dbl)
                  n125 = local read "拟合起点"() -> (w329:i32)
                  n126 = local read "拟合终点"() -> (w331:i32)
                  n127 = call <vilib>:"Median Filter.vi"("left rank"=6, "X"=w319) -> ("Filtered X"=w318:dbl[])  [unwired: 8 in, 1 out]
                  n128 = Build Array(w321, w314, 0.0 ("元素")) -> (w320:dbl[])
                  n129 = Subtract(x=w331, y=w329) -> (x-y=w328:i32)
                  n130 = call "Convert to Dynamic Data"("Array"=w322) -> ("Dynamic Data Type"=w350:dynamicdata)  [unwired: 3 in]
                  n131 = call "Convert to Dynamic Data2"("Array"=w319) -> ("Dynamic Data Type"=w349:dynamicdata)  [unwired: 3 in]
                  n132 = Array Subset(array=w322, index=w329, length=w328) -> (w327:dbl[])
                  n133 = call "Build XY Graph"("Y Input"=w349, "X Input"=w350) -> ("XY Graph"=→"Spectrum":cluster{"Y":dbl[], "Y":dbl[]}[])  [unwired: 8 in, 1 out]
                  n134 = call "转换至动态数据4"("Array"=w327) -> ("Dynamic Data Type"=w347:dynamicdata)  [unwired: 3 in]
                  n135 = In Range and Coerce(upper limit="滤波阈值", x=w318, lower limit=-100.0) -> (In Range?=w334:bool[])  [unwired: 1 out]
                  "范围内？" <- w334
                  n136 = Not(x=w334) -> (.not. x?=w333:bool[])
                  n137 = Or Array Elements(Boolean array=w333) -> (logical OR=w336:bool)
                  n138 = local read "X Pixels:"() -> (w335:i32)
                  n139 = local read "波长范围"() -> (w323:dbl[])
                  n140 = local read "滤波阈值"() -> (w332:dbl)
                  n141 = case shown="真" w336 {
                    tunnel: w335 -> [_ w386]
                    tunnel: w318 -> [w382 w385]
                    tunnel: [w382 w384] -> w312
                    tunnel: w332 -> [_ w383]
                    frame False {
                    }
                    frame True {
                      n142 = for {
                        N: w386 -> [_]
                        tunnel: w385 -> [w390] mode=indexing
                        tunnel: [w389] -> w384 mode=indexing
                        shift-right: [w389] -> _
                        shift-left: _ -> [w388]
                        tunnel: w383 -> [w387]
                        n143 = Greater?(x=w390, y=w387) -> (0:w392:bool)
                        n144 = Less?(x=w390, y=-100.0) -> (x < y?=w393:bool)
                        n145 = Or(x=w392, y=w393) -> (x .or. y?=w391:bool)
                        n146 = case shown="真" w391 {
                          tunnel: w390 -> [w395 _]
                          tunnel: [w395 w397] -> w389
                          tunnel: w388 -> [_ w398]
                          frame False {
                          }
                          frame True {
                            n147 = call <vilib>:"Median Filter PtByPt.vi"("rank"=5, "x"=w398) -> ("Filtered x"=w397:dbl)  [unwired: 2 in, 1 out]
                          }
                        }
                      }
                    }
                  }
                  n148 = Array Subset(array=w312, index=w329, length=w328) -> (w330:dbl[])
                  n149 = call "转换至动态数据3"("Array"=w330) -> ("Dynamic Data Type"=w348:dynamicdata)  [unwired: 3 in]
                  n150 = call "曲线拟合"("Locations"=w347, "Signals"=w348) -> ("best fit"=w352:dynamicdata, "non-linear coefficients"=w351:dynamicdata)  [unwired: 5 in, 3 out]
                  n151 = call "从动态数据转换"("Dynamic Data Type"=w351) -> ("Array"=w344:dbl[])  [unwired: 3 in]
                  "拟合参数" <- w344
                  n152 = call "从动态数据转换2"("Dynamic Data Type"=w352) -> ("Array"=w313:dbl[])  [unwired: 3 in]
                  n153 = Build Array(w322, w318, w313, w344, w320) -> (w381:dbl[][])
                  n154 = call-poly <vilib>:"Write Delimited Spreadsheet.vi"("file path (dialog if empty)"=w378, "format (%.3f)"="%.16f", "2D data"=w381, "append to file? (new file:F)"=TRUE ("append to file? (F)"), "transpose? (no:F)"=TRUE ("transpose? (F)")) -> ()  [unwired: 9 in, 2 out]
                  n155 = Index Array(array=w344, index #1=0 ("索引"), index #2=1 ("索引")) -> (element #1=→"xc":dbl, element #2=w316:dbl)
                  "w" <- w316
                  n156 = Bundle("波长范围"=w323, "Filtered X"=w312) -> (w326:cluster{"波长范围 ":dbl[], "Filtered X":dbl[]})  [unwired: 1 in]
                  n157 = Bundle(w327, "Array"=w313) -> (w325:cluster{dbl[], "Array":dbl[]})  [unwired: 1 in]
                  n158 = Array Max & Min(array=w313) -> (max value=w310:dbl)  [unwired: 3 out]
                  "拟合峰值" <- w310
                  n159 = Array Max & Min(array=w312) -> (max value=w311:dbl)  [unwired: 3 out]
                  "原始峰值" <- w311
                  n160 = Build Array(w326, w325) -> (w324:cluster{"波长范围 ":dbl[], "Array":dbl[]}[])
                  n161 = local write "best fit"(w324) -> ()
                }
                frame #7 {
                  n162 = Open Python Session(python version="3.9" ("Python version")) -> (session out=w409:refnum<k35>, error out=w408:errorcluster)  [unwired: 2 in]
                  n163 = node(w409, path "D:/desktop/train/newpro_wan.py" ("module path"), "changexls2xlsx" ("function name"), w408, w403) -> (w405:refnum<k35>, w404:errorcluster)  [unwired: 3 in, 2 out]
                  n164 = Close Python Session(session in=w405, error in=w404) -> ()  [unwired: 1 out]
                }
                frame #8 {
                  n165 = flat-sequence {
                    tunnel: w414 -> [w423]
                    tunnel: w413 -> [w422]
                    tunnel: [w418] -> w412
                    tunnel: [w417] -> w411
                    frame #0 {
                      n166 = local read "channel输出口"() -> (w416:i32)
                      n167 = case shown="1" w416 {
                        tunnel: [1 0] -> w415
                        frame 0, Default {
                        }
                        frame 1 {
                        }
                      }
                      n168 = local write "Output 2"(TRUE ("布尔")) -> ()
                      n169 = Pick Line(multi-line string=":OUTP1 ON\n:OUTP2 ON" ("write buffer"), line index=w415) -> (output string=w419:string)  [unwired: 1 in]
                      n170 = VISA Write(VISA resource name=w423, write buffer=w419, error in (no error)=w422) -> (VISA resource name out=w418:refnum<visa-resource-name>, error out=w417:errorcluster)  [unwired: 1 out]
                    }
                  }
                }
                frame #9 {
                  w426 = " \u0001\u0000¡"  # Channel
                  n171 = Concatenate Strings(w426, "\r") -> (w432:string)
                  n172 = VISA Write(VISA resource name=w428, write buffer=w432, error in (no error)=w431) -> (VISA resource name out=w430:refnum<visa-resource-name>, error out=w429:errorcluster)  [unwired: 1 out]
                  n173 = local write "照明光"(TRUE ("照明光")) -> ()
                }
                frame #10 {
                  n174 = Wait (ms)(milliseconds to wait=1200) -> ()  [unwired: 1 out]
                }
                frame #11 {
                  n175 = Greater Or Equal?(x=w437, y=1) -> (x >= y?=w438:bool)
                  n176 = case shown="真" w438 {
                    tunnel: w440 -> [_ w446]
                    tunnel: w439 -> [_ w447]
                    tunnel: w435 -> [w441 w448]
                    frame False {
                      n177 = local write "w0"(w441) -> ()
                    }
                    frame True {
                      n178 = local read "Δw1>C"() -> (w445:bool)
                      n179 = case shown="真" w445 {
                        tunnel: w448 -> [w467 w487]
                        tunnel: w447 -> [w457 _]
                        tunnel: w446 -> [w458 _]
                        frame False {
                          # "判断Δw突变位置并记录当前θ值"
                          # "根据θ变化速度改变开光时间"
                          n180 = local read "w0"() -> (w465:dbl)
                          n181 = Subtract(x=w458, y=w457) -> (x-y=w460:dbl)
                          n182 = local read "开光时间/ms"() -> (w463:u32)
                          n183 = Subtract(x=w465, y=w467) -> (x-y=w470:dbl)
                          n184 = Absolute Value(x=w460) -> (abs(x)=w462:dbl)
                          n185 = Absolute Value(x=w470) -> (abs(x)=w468:dbl)
                          n186 = Greater Or Equal?(x=w462, y="角度判断上限") -> (x >= y?=w461:bool)
                          n187 = Greater Or Equal?(x=w468, y="C=w-w0") -> (x >= y?=w466:bool)
                          n188 = case shown="真" w466 {
                            tunnel: w457 -> [_ w485]
                            frame False {
                              w483 = FALSE ("Δw1>C")
                              n189 = local write "Δw1>C"(w483) -> ()
                              n190 = local write "Δw2>C"(w483) -> ()
                            }
                            frame True {
                              "θi" <- w485
                              "Δw1>C" <- TRUE ("布尔")
                            }
                          }
                          n191 = case shown="假" w461 {
                            tunnel: w462 -> [w475 _]
                            tunnel: w463 -> [w472 w482]
                            tunnel: [w471 w480] -> w464
                            frame False {
                              n192 = Less Or Equal?(x=w475, y="角度判断下限") -> (x <= y?=w473:bool)
                              n193 = case shown="真" w473 {
                                tunnel: w472 -> [w476 w479]
                                tunnel: [w476 w478] -> w471
                                frame False {
                                }
                                frame True {
                                n194 = Multiply(x=w479, y="角度倍乘系数") -> (x*y=w478:dbl)
                                }
                              }
                            }
                            frame True {
                              n195 = Divide(x=w482, y=1.6) -> (x/y=w480:dbl)
                            }
                          }
                          n196 = local write "开光时间/ms"(w464) -> ()
                        }
                        frame True {
                          # "再次判断Δw，排除坏点影响"
                          n197 = local read "Δw2>C"() -> (w486:bool)
                          n198 = case shown="假" w486 {
                            tunnel: w487 -> [w492 _]
                            frame False {
                              n199 = local read "C=w-w0"() -> (w489:dbl)
                              n200 = local read "w0"() -> (w493:dbl)
                              n201 = Subtract(x=w493, y=w492) -> (x-y=w495:dbl)
                              n202 = Absolute Value(x=w495) -> (abs(x)=w494:dbl)
                              n203 = Add(x=w489, y=0) -> (x+y=w488:dbl)
                              n204 = Greater Or Equal?(x=w494, y=w488) -> (x >= y?=w491:bool)
                              n205 = case shown="真" w491 {
                                frame False {
                                n206 = local write "θi"(0.0 ("θi")) -> ()
                                n207 = local write "Δw1>C"(FALSE ("Δw1>C")) -> ()
                                }
                                frame True {
                                "Δw2>C" <- TRUE
                                }
                              }
                            }
                            frame True {
                            }
                          }
                        }
                      }
                      n208 = local read "Δw1>C"() -> (w443:bool)
                      n209 = local read "Δw2>C"() -> (w444:bool)
                      n210 = And(x=w443, y=w444) -> (x .and. y?=w442:bool)
                      n211 = case shown="假" w442 {
                        tunnel: w446 -> [_ w449]
                        frame False {
                        }
                        frame True {
                          # "4°后重置指示灯状态"
                          n212 = local read "θi"() -> (w453:dbl)
                          n213 = Subtract(x=w449, y=w453) -> (x-y=w454:dbl)
                          n214 = Absolute Value(x=w454) -> (abs(x)=w452:dbl)
                          n215 = Greater?(x=w452, y=4.0) -> (0:w450:bool)
                          n216 = case shown="真" w450 {
                            frame False {
                            }
                            frame True {
                              w455 = FALSE ("Δw1>C")
                              n217 = local write "Δw1>C"(w455) -> ()
                              n218 = local write "Δw2>C"(w455) -> ()
                              n219 = local write "θi"(0.0 ("θ")) -> ()
                            }
                          }
                        }
                      }
                    }
                  }
                }
                frame #12 {
                  n220 = local write "正在测量"(FALSE) -> ()
                }
              }
              n221 = Build Array(w148, w147, w146, w145, w141) -> (w139:dbl[])
              n222 = local read "结果展示"() -> (w138:dbl[][])
              n223 = Insert Into Array(array=w138, new element=w139) -> (→"结果展示":dbl[][])  [unwired: 2 in]
            }
            n224 = Path To String(path=w101) -> (string=w109:string)
            n225 = Concatenate Strings(w109, "循环汇总" ("字符串"), ".xls" ("字符串")) -> (w97:string)
            n226 = VISA Close(VISA resource name=w124, error in (no error)=w123) -> (error out=→"output control error":errorcluster)
            n227 = VISA Close(VISA resource name=w127, error in (no error)=w126) -> (error out=→"照明光error out":errorcluster)
            n228 = String To Path(string=w97) -> (path=w108:path)
            n229 = local write "结果展示"(dbl[][] [] ("结果展示")) -> ()
            n230 = call-poly <vilib>:"Write Delimited Spreadsheet.vi"("file path (dialog if empty)"=w108, "format (%.3f)"="%.16f", "2D data"=w104, "append to file? (new file:F)"=TRUE ("append to file? (F)"), "transpose? (no:F)"=FALSE ("transpose? (F)")) -> ()  [unwired: 9 in, 2 out]
          }
          frame #1 {
            n231 = Open Python Session(python version="3.9" ("Python version")) -> (session out=w506:refnum<k35>, error out=w505:errorcluster)  [unwired: 2 in]
            n232 = node(w506, path "D:/desktop/train/newpro_wan.py" ("module path"), "changexls2xlsx" ("function name"), w505, w500) -> (w502:refnum<k35>, w501:errorcluster)  [unwired: 3 in, 2 out]
            n233 = Close Python Session(session in=w502, error in=w501) -> ()  [unwired: 1 out]
          }
        }
      }
    }
    n234 = event shown="[1] \"低电平持续输出\": 值改变" {
      selector: _ -> [_ _]
      dyn-events: _ -> [_ _]
      timeout: u32 0 ("Time") -> [_ _]
      tunnel: "低电平持续输出" -> [_ w537]
      event Timeout {
        n235 = event-data() -> ()  [unwired: 1 in, 2 out]
      }
      event "低电平持续输出": Value Change {
        w541 = " :SOUR1\n :SOUR2"  # Channel
        n236 = event-data() -> ()  [unwired: 1 in, 6 out]
        n237 = local read "channel输出口"() -> (w542:i32)
        n238 = Pick Line(multi-line string=w541, line index=w542) -> (output string=w540:string)  [unwired: 1 in]
        n239 = local read "VISA 信号发生器"() -> (w545:refnum<visa-resource-name>)
        n240 = VISA Open(VISA resource name=w545) -> (VISA resource name=w544:refnum<visa-resource-name>, error out=w543:errorcluster)  [unwired: 4 in]
        n241 = stacked-sequence {
          seq-local: [w551 _ _ _ _ _ _ _ _ _ _ _ _] -> [_ _ w566 _ _ _ _ _ _ _ _ _ _]
          seq-local: [w550 _ _ _ _ _ _ _ _ _ _ _ _] -> [_ _ w565 _ _ _ _ _ _ _ _ _ _]
          seq-local: [_ _ w564 _ _ _ _ _ _ _ _ _ _] -> [_ _ _ _ w569 _ _ _ _ _ _ _ _]
          seq-local: [_ _ w563 _ _ _ _ _ _ _ _ _ _] -> [_ _ _ _ w570 _ _ _ _ _ _ _ _]
          seq-local: [_ _ _ _ w578 _ _ _ _ _ _ _ _] -> [_ _ _ _ _ _ w589 _ _ _ _ _ _]
          seq-local: [_ _ _ _ w577 _ _ _ _ _ _ _ _] -> [_ _ _ _ _ _ w588 _ _ _ _ _ _]
          seq-local: [_ _ _ _ _ _ w582 _ _ _ _ _ _] -> [_ _ _ _ _ _ _ _ w592 _ _ _ _]
          seq-local: [_ _ _ _ _ _ w581 _ _ _ _ _ _] -> [_ _ _ _ _ _ _ _ w591 _ _ _ _]
          seq-local: [_ _ _ _ _ _ _ _ w595 _ _ _ _] -> [_ _ _ _ _ _ _ _ _ _ w606 _ _]
          seq-local: [_ _ _ _ _ _ _ _ w594 _ _ _ _] -> [_ _ _ _ _ _ _ _ _ _ w605 _ _]
          seq-local: [_ _ _ _ _ _ _ _ _ _ w603 _ _] -> [_ _ _ _ _ _ _ _ _ _ _ _ w620]
          seq-local: [_ _ _ _ _ _ _ _ _ _ w602 _ _] -> [_ _ _ _ _ _ _ _ _ _ _ _ w619]
          tunnel: w544 -> [w556 _ _ _ _ _ _ _ _ _ _ _ _]
          tunnel: w543 -> [w549 _ _ _ _ _ _ _ _ _ _ _ _]
          tunnel: w540 -> [w548 _ w562 _ w575 _ w586 _ w596 _ w609 _ _]
          tunnel: [_ _ _ _ _ _ _ _ _ _ _ _ w618] -> w539
          tunnel: [_ _ _ _ _ _ _ _ _ _ _ _ w616] -> w538
          tunnel: w537 -> [_ _ _ _ _ _ _ _ _ _ _ _ w617]
          frame #0 {
            w553 = " PULSe"  # Function Command
            n242 = local read "输出信号波形"() -> (w547:u16)
            n243 = Concatenate Strings(w548, ":FUNC" ("string (\"\")")) -> (w554:string)
            n244 = Pick Line(string ("")=w554, multi-line string=w553, line index=w547) -> (output string=w552:string)
            n245 = VISA Write(VISA resource name=w556, write buffer=w552, error in (no error)=w549) -> (VISA resource name out=w551:refnum<visa-resource-name>, error out=w550:errorcluster)  [unwired: 1 out]
          }
          frame #1 {
            n246 = Wait (ms)(milliseconds to wait=u32 150) -> ()  [unwired: 1 out]
          }
          frame #2 {
            n247 = Number To Fractional String(use system decimal point (T)=TRUE ("使用系统小数点(T)"), number=1.0 ("数字")) -> (F-format string=w560:string)  [unwired: 2 in]
            n248 = Concatenate Strings ("连接字符串")(w562, ":VOLTage：HIGH ", w560) -> (w559:string)
            n249 = VISA Write(VISA resource name=w566, write buffer=w559, error in (no error)=w565) -> (VISA resource name out=w564:refnum<visa-resource-name>, error out=w563:errorcluster)  [unwired: 1 out]
          }
          frame #3 {
            n250 = Wait (ms)(milliseconds to wait=u32 150) -> ()  [unwired: 1 out]
          }
          frame #4 {
            # "1 电压偏置"
            n251 = Number To Fractional String(use system decimal point (T)=TRUE ("使用系统小数点(T)"), number=0.0 ("数字")) -> (F-format string=w573:string)  [unwired: 2 in]
            n252 = Concatenate Strings(w575, ":VOLTage:LOW ", w573) -> (w574:string)
            n253 = VISA Write(VISA resource name=w569, write buffer=w574, error in (no error)=w570) -> (VISA resource name out=w578:refnum<visa-resource-name>, error out=w577:errorcluster)  [unwired: 1 out]
          }
          frame #5 {
            n254 = Wait (ms)(milliseconds to wait=u32 150) -> ()  [unwired: 1 out]
          }
          frame #6 {
            n255 = local read "channel输出口"() -> (w584:i32)
            n256 = Pick Line(multi-line string=":OUTP1:IMPedance \n:OUTP2:IMPedance " ("write buffer"), line index=w584) -> (output string=w583:string)  [unwired: 1 in]
            n257 = Concatenate Strings ("连接字符串")(w586, w583, "INFINITY") -> (w587:string)
            n258 = VISA Write(VISA resource name=w589, write buffer=w587, error in (no error)=w588) -> (VISA resource name out=w582:refnum<visa-resource-name>, error out=w581:errorcluster)  [unwired: 1 out]
          }
          frame #7 {
            n259 = Wait (ms)(milliseconds to wait=u32 150) -> ()  [unwired: 1 out]
          }
          frame #8 {
            n260 = Number To Fractional String(use system decimal point (T)=TRUE ("使用系统小数点(T)"), number=0.0 ("数字")) -> (F-format string=w599:string)  [unwired: 2 in]
            n261 = Concatenate Strings(w596, ":PULSe:DELay ", w599) -> (w597:string)
            n262 = VISA Write(VISA resource name=w592, write buffer=w597, error in (no error)=w591) -> (VISA resource name out=w595:refnum<visa-resource-name>, error out=w594:errorcluster)  [unwired: 1 out]
          }
          frame #9 {
            n263 = Wait (ms)(milliseconds to wait=u32 150) -> ()  [unwired: 1 out]
          }
          frame #10 {
            w610 = ":LEADing\n:TRAiling "  # Channel
            w614 = ":PULSe:TRANsition"  # VOLTage:Offset
            n264 = local read "上升下降沿"() -> (w611:i32)
            n265 = Pick Line(multi-line string=w610, line index=w611) -> (output string=w607:string)  [unwired: 1 in]
            n266 = Number To Fractional String(use system decimal point (T)=TRUE ("使用系统小数点(T)"), number=0.0 ("数字")) -> (F-format string=w608:string)  [unwired: 2 in]
            n267 = Concatenate Strings(w609, w614, w607, w608) -> (w612:string)
            n268 = VISA Write(VISA resource name=w606, write buffer=w612, error in (no error)=w605) -> (VISA resource name out=w603:refnum<visa-resource-name>, error out=w602:errorcluster)  [unwired: 1 out]
          }
          frame #11 {
            n269 = Wait (ms)(milliseconds to wait=u32 150) -> ()  [unwired: 1 out]
          }
          frame #12 {
            n270 = case shown="假" w617 {
              tunnel: w620 -> [w628 w629]
              tunnel: [w627 w636] -> w616
              tunnel: w619 -> [w626 w634]
              tunnel: [w625 w635] -> w618
              frame True {
                n271 = local write "Output"(TRUE ("布尔")) -> ()
                n272 = local read "channel输出口"() -> (w622:i32)
                n273 = Pick Line(multi-line string=":OUTP1 ON\n:OUTP2 ON" ("write buffer"), line index=w622) -> (output string=w621:string)  [unwired: 1 in]
                n274 = VISA Write(VISA resource name=w628, write buffer=w621, error in (no error)=w626) -> (VISA resource name out=w625:refnum<visa-resource-name>, error out=w627:errorcluster)  [unwired: 1 out]
              }
              frame False {
                n275 = local read "channel输出口"() -> (w631:i32)
                n276 = Pick Line(multi-line string=":OUTP1 OFF\n:OUTP2 OFF" ("write buffer"), line index=w631) -> (output string=w630:string)  [unwired: 1 in]
                n277 = VISA Write(VISA resource name=w629, write buffer=w630, error in (no error)=w634) -> (VISA resource name out=w635:refnum<visa-resource-name>, error out=w636:errorcluster)  [unwired: 1 out]
                n278 = local write "Output"(FALSE ("布尔")) -> ()
              }
            }
          }
        }
        n279 = VISA Close(VISA resource name=w539, error in (no error)=w538) -> (error out=→"output control error  4":errorcluster)
      }
    }
    n280 = event shown="[1] \"Enable\": 值改变" {
      selector: _ -> [_ _]
      dyn-events: _ -> [_ _]
      timeout: u32 0 ("Time") -> [_ _]
      tunnel: "Enable" -> [_ w512]
      event Timeout {
        n281 = event-data() -> ()  [unwired: 1 in, 2 out]
      }
      event "Enable": Value Change {
        n282 = event-data() -> ()  [unwired: 1 in, 6 out]
        n283 = local read "VISA 信号发生器"() -> (w508:refnum<visa-resource-name>)
        n284 = VISA Open(VISA resource name=w508) -> (VISA resource name=w511:refnum<visa-resource-name>, error out=w514:errorcluster)  [unwired: 4 in]
        n285 = stacked-sequence {
          tunnel: w512 -> [w519 _]
          tunnel: w514 -> [w518 _]
          tunnel: w511 -> [w517 _]
          tunnel: [w516 _] -> w510
          tunnel: [w515 _] -> w509
          frame #0 {
            n286 = case shown="真" w519 {
              tunnel: w517 -> [w527 w535]
              tunnel: [w526 w534] -> w515
              tunnel: w518 -> [w525 w532]
              tunnel: [w524 w533] -> w516
              frame True {
                n287 = local write "Output"(TRUE ("布尔")) -> ()
                n288 = local read "channel输出口"() -> (w521:i32)
                n289 = Pick Line(multi-line string=":OUTP1 ON\n:OUTP2 ON" ("write buffer"), line index=w521) -> (output string=w520:string)  [unwired: 1 in]
                n290 = VISA Write(VISA resource name=w527, write buffer=w520, error in (no error)=w525) -> (VISA resource name out=w524:refnum<visa-resource-name>, error out=w526:errorcluster)  [unwired: 1 out]
              }
              frame False {
                n291 = local read "channel输出口"() -> (w529:i32)
                n292 = Pick Line(multi-line string=":OUTP1 OFF\n:OUTP2 OFF" ("write buffer"), line index=w529) -> (output string=w528:string)  [unwired: 1 in]
                n293 = VISA Write(VISA resource name=w535, write buffer=w528, error in (no error)=w532) -> (VISA resource name out=w533:refnum<visa-resource-name>, error out=w534:errorcluster)  [unwired: 1 out]
                n294 = local write "Output"(FALSE ("布尔")) -> ()
              }
            }
          }
          frame #1 {
            n295 = Wait (ms)(milliseconds to wait=u32 150) -> ()  [unwired: 1 out]
          }
        }
        n296 = VISA Close(VISA resource name=w510, error in (no error)=w509) -> (error out=→"output control error  5":errorcluster)
      }
    }
    n297 = event shown="[1] \"Enable 2\": 值改变" {
      selector: _ -> [_ _]
      dyn-events: _ -> [_ _]
      timeout: u32 0 ("Time") -> [_ _]
      tunnel: "Enable 2" -> [_ w27]
      event Timeout {
        n298 = event-data() -> ()  [unwired: 1 in, 2 out]
      }
      event "Enable 2": Value Change {
        n299 = event-data() -> ()  [unwired: 1 in, 6 out]
        n300 = Not(x=w27) -> (.not. x?=w26:bool)
        n301 = local read "VISA 信号发生器"() -> (w28:refnum<visa-resource-name>)
        n302 = VISA Open(VISA resource name=w28) -> (VISA resource name=w31:refnum<visa-resource-name>, error out=w32:errorcluster)  [unwired: 4 in]
        n303 = stacked-sequence {
          tunnel: w26 -> [w37 _]
          tunnel: w32 -> [w36 _]
          tunnel: w31 -> [w35 _]
          tunnel: [w34 _] -> w30
          tunnel: [w33 _] -> w29
          frame #0 {
            n304 = case shown="真" w37 {
              tunnel: w35 -> [w46 w57]
              tunnel: [w45 w56] -> w33
              tunnel: w36 -> [w44 w54]
              tunnel: [w43 w55] -> w34
              frame True {
                n305 = local read "channel输出口"() -> (w39:i32)
                n306 = local write "Output 2"(FALSE ("布尔")) -> ()
                n307 = case shown="1" w39 {
                  tunnel: [1 0] -> w38
                  frame 0, Default {
                  }
                  frame 1 {
                  }
                }
                n308 = Pick Line(multi-line string=":OUTP1 ON\n:OUTP2 ON" ("write buffer"), line index=w38) -> (output string=w40:string)  [unwired: 1 in]
                n309 = VISA Write(VISA resource name=w46, write buffer=w40, error in (no error)=w44) -> (VISA resource name out=w43:refnum<visa-resource-name>, error out=w45:errorcluster)  [unwired: 1 out]
              }
              frame False {
                n310 = local read "channel输出口"() -> (w50:i32)
                n311 = case shown="1" w50 {
                  tunnel: [1 0] -> w49
                  frame 0, Default {
                  }
                  frame 1 {
                  }
                }
                n312 = Pick Line(multi-line string=":OUTP1 OFF\n:OUTP2 OFF" ("write buffer"), line index=w49) -> (output string=w51:string)  [unwired: 1 in]
                n313 = VISA Write(VISA resource name=w57, write buffer=w51, error in (no error)=w54) -> (VISA resource name out=w55:refnum<visa-resource-name>, error out=w56:errorcluster)  [unwired: 1 out]
                n314 = local write "Output 2"(TRUE ("布尔")) -> ()
              }
            }
          }
          frame #1 {
            n315 = Wait (ms)(milliseconds to wait=u32 150) -> ()  [unwired: 1 out]
          }
        }
        n316 = VISA Close(VISA resource name=w30, error in (no error)=w29) -> ()  [unwired: 1 out]
      }
    }
    n317 = case shown="真" "设置参数" {
      frame False {
      }
      frame True {
        w643 = " :SOUR1\n :SOUR2"  # Channel
        n318 = local read "VISA 信号发生器"() -> (w645:refnum<visa-resource-name>)
        n319 = local read "channel输出口"() -> (w644:i32)
        n320 = case shown="1" w644 {
          tunnel: [1 0] -> w637
          frame 0, Default {
          }
          frame 1 {
          }
        }
        n321 = VISA Open(VISA resource name=w645) -> (VISA resource name=w648:refnum<visa-resource-name>, error out=w649:errorcluster)  [unwired: 4 in]
        n322 = Pick Line(multi-line string=w643, line index=w637) -> (output string=w638:string)  [unwired: 1 in]
        n323 = Pick Line(multi-line string=w643, line index=w644) -> (output string=w646:string)  [unwired: 1 in]
        n324 = stacked-sequence {
          seq-local: [w745 _ _ _ _ _ _ _ _ _ _ _ _ _ _] -> [_ _ w760 _ _ _ _ _ _ _ _ _ _ _ _]
          seq-local: [w744 _ _ _ _ _ _ _ _ _ _ _ _ _ _] -> [_ _ w759 _ _ _ _ _ _ _ w798 _ _ _ _]
          seq-local: [_ _ w758 _ _ _ _ _ _ _ _ _ _ _ _] -> [_ _ _ _ w769 _ _ _ _ _ _ _ _ _ _]
          seq-local: [_ _ w757 _ _ _ _ _ _ _ _ _ _ _ _] -> [_ _ _ _ w768 _ _ _ _ _ _ _ _ _ _]
          seq-local: [_ _ _ _ w767 _ _ _ _ _ _ _ _ _ _] -> [_ _ _ _ _ _ w775 _ _ _ _ _ _ _ _]
          seq-local: [_ _ _ _ w764 _ _ _ _ _ _ _ _ _ _] -> [_ _ _ _ _ _ w774 _ _ _ _ _ _ _ _]
          seq-local: [_ _ _ _ _ _ w782 _ _ _ _ _ _ _ _] -> [_ _ _ _ _ _ _ _ w793 _ _ _ _ _ _]
          seq-local: [_ _ _ _ _ _ w781 _ _ _ _ _ _ _ _] -> [_ _ _ _ _ _ _ _ w792 _ _ _ _ _ _]
          seq-local: [_ _ _ _ _ _ _ _ w786 _ _ _ _ _ _] -> [_ _ _ _ _ _ _ _ _ _ w799 _ _ _ _]
          seq-local: [_ _ _ _ _ _ _ _ w785 _ _ _ _ _ _] -> [_ _ _ _ _ _ _ _ _ _ _ _ _ _ _]
          seq-local: [_ _ _ _ _ _ _ _ _ _ w795 _ _ _ _] -> [_ _ _ _ _ _ _ _ _ _ _ _ w809 _ _]
          seq-local: [_ _ _ _ _ _ _ _ _ _ w796 _ _ _ _] -> [_ _ _ _ _ _ _ _ _ _ _ _ w808 _ _]
          seq-local: [_ _ _ _ _ _ _ _ _ _ _ _ w807 _ _] -> [_ _ _ _ _ _ _ _ _ _ _ _ _ _ w820]
          seq-local: [_ _ _ _ _ _ _ _ _ _ _ _ w806 _ _] -> [_ _ _ _ _ _ _ _ _ _ _ _ _ _ w819]
          tunnel: w648 -> [w750 _ _ _ _ _ _ _ _ _ _ _ _ _ _]
          tunnel: w649 -> [w743 _ _ _ _ _ _ _ _ _ _ _ _ _ _]
          tunnel: w646 -> [w742 _ w756 _ w763 _ w779 _ w790 _ w800 _ w810 _ w823]
          tunnel: [_ _ _ _ _ _ _ _ _ _ _ _ _ _ w818] -> w642
          tunnel: [_ _ _ _ _ _ _ _ _ _ _ _ _ _ w817] -> w641
          frame #0 {
            w747 = " PULSe"  # Function Command
            n325 = local read "输出信号波形"() -> (w741:u16)
            n326 = Concatenate Strings(w742, ":FUNC" ("string (\"\")")) -> (w748:string)
            n327 = Pick Line(string ("")=w748, multi-line string=w747, line index=w741) -> (output string=w746:string)
            n328 = VISA Write(VISA resource name=w750, write buffer=w746, error in (no error)=w743) -> (VISA resource name out=w745:refnum<visa-resource-name>, error out=w744:errorcluster)  [unwired: 1 out]
          }
          frame #1 {
            n329 = Wait (ms)(milliseconds to wait=u32 150) -> ()  [unwired: 1 out]
          }
          frame #2 {
            n330 = Number To Fractional String(use system decimal point (T)=TRUE ("使用系统小数点(T)"), number="低电平/V") -> (F-format string=w754:string)  [unwired: 2 in]
            n331 = Concatenate Strings ("连接字符串")(w756, ":VOLTage:LOW ", w754) -> (w753:string)
            n332 = VISA Write(VISA resource name=w760, write buffer=w753, error in (no error)=w759) -> (VISA resource name out=w758:refnum<visa-resource-name>, error out=w757:errorcluster)  [unwired: 1 out]
          }
          frame #3 {
            n333 = Wait (ms)(milliseconds to wait=u32 150) -> ()  [unwired: 1 out]
          }
          frame #4 {
            # "1 频率"
            n334 = Concatenate Strings(w763, ":FREQ ") -> (w770:string)
            n335 = Format Into String ("格式化写入字符串")(initial string=w770, "频率/Hz") -> (resulting string=w771:string)  [unwired: 2 in, 1 out]
            n336 = VISA Write(VISA resource name=w769, write buffer=w771, error in (no error)=w768) -> (VISA resource name out=w767:refnum<visa-resource-name>, error out=w764:errorcluster)  [unwired: 1 out]
          }
          frame #5 {
            n337 = Wait (ms)(milliseconds to wait=u32 150) -> ()  [unwired: 1 out]
          }
          frame #6 {
            n338 = Number To Fractional String(use system decimal point (T)=TRUE ("使用系统小数点(T)"), number="高电平/V") -> (F-format string=w776:string)  [unwired: 2 in]
            n339 = Concatenate Strings(w779, ":VOLTage:HIGH ", w776) -> (w778:string)
            n340 = VISA Write(VISA resource name=w775, write buffer=w778, error in (no error)=w774) -> (VISA resource name out=w782:refnum<visa-resource-name>, error out=w781:errorcluster)  [unwired: 1 out]
          }
          frame #7 {
            n341 = Wait (ms)(milliseconds to wait=u32 150) -> ()  [unwired: 1 out]
          }
          frame #8 {
            n342 = local read "channel输出口"() -> (w788:i32)
            n343 = Pick Line(multi-line string=":OUTP1:IMPedance \n:OUTP2:IMPedance " ("write buffer"), line index=w788) -> (output string=w787:string)  [unwired: 1 in]
            n344 = Concatenate Strings ("连接字符串")(w790, w787, "INFINITY") -> (w791:string)
            n345 = VISA Write(VISA resource name=w793, write buffer=w791, error in (no error)=w792) -> (VISA resource name out=w786:refnum<visa-resource-name>, error out=w785:errorcluster)  [unwired: 1 out]
          }
          frame #9 {
            n346 = Wait (ms)(milliseconds to wait=u32 150) -> ()  [unwired: 1 out]
          }
          frame #10 {
            n347 = Number To Fractional String(use system decimal point (T)=TRUE ("使用系统小数点(T)"), number="占空比/%") -> (F-format string=w802:string)  [unwired: 2 in]
            n348 = Concatenate Strings(w800, ":PULSe:DCYCle ", w802) -> (w797:string)
            n349 = VISA Write(VISA resource name=w799, write buffer=w797, error in (no error)=w798) -> (VISA resource name out=w795:refnum<visa-resource-name>, error out=w796:errorcluster)  [unwired: 1 out]
          }
          frame #11 {
            n350 = Wait (ms)(milliseconds to wait=u32 150) -> ()  [unwired: 1 out]
          }
          frame #12 {
            n351 = Number To Fractional String(use system decimal point (T)=TRUE ("使用系统小数点(T)"), number="延时/s") -> (F-format string=w813:string)  [unwired: 2 in]
            n352 = Concatenate Strings(w810, ":PULSe:DELay ", w813) -> (w811:string)
            n353 = VISA Write(VISA resource name=w809, write buffer=w811, error in (no error)=w808) -> (VISA resource name out=w807:refnum<visa-resource-name>, error out=w806:errorcluster)  [unwired: 1 out]
          }
          frame #13 {
            n354 = Wait (ms)(milliseconds to wait=u32 150) -> ()  [unwired: 1 out]
          }
          frame #14 {
            w824 = ":LEADing\n:TRAiling "  # Channel
            w829 = ":PULSe:TRANsition"  # VOLTage:Offset
            n355 = local read "上升下降沿"() -> (w825:i32)
            n356 = Pick Line(multi-line string=w824, line index=w825) -> (output string=w821:string)  [unwired: 1 in]
            n357 = Number To Fractional String(use system decimal point (T)=TRUE ("使用系统小数点(T)"), number="上升下降沿/s") -> (F-format string=w822:string)  [unwired: 2 in]
            n358 = Concatenate Strings(w823, w829, w821, w822) -> (w826:string)
            n359 = VISA Write(VISA resource name=w820, write buffer=w826, error in (no error)=w819) -> (VISA resource name out=w818:refnum<visa-resource-name>, error out=w817:errorcluster)  [unwired: 1 out]
          }
        }
        n360 = stacked-sequence {
          seq-local: [w656 _ _ _ _ _ _ _ _ _ _ _ _ _ _] -> [_ _ w671 _ _ _ _ _ _ _ _ _ _ _ _]
          seq-local: [w655 _ _ _ _ _ _ _ _ _ _ _ _ _ _] -> [_ _ w670 _ _ _ _ _ _ _ w709 _ _ _ _]
          seq-local: [_ _ w669 _ _ _ _ _ _ _ _ _ _ _ _] -> [_ _ _ _ w680 _ _ _ _ _ _ _ _ _ _]
          seq-local: [_ _ w668 _ _ _ _ _ _ _ _ _ _ _ _] -> [_ _ _ _ w679 _ _ _ _ _ _ _ _ _ _]
          seq-local: [_ _ _ _ w678 _ _ _ _ _ _ _ _ _ _] -> [_ _ _ _ _ _ w686 _ _ _ _ _ _ _ _]
          seq-local: [_ _ _ _ w675 _ _ _ _ _ _ _ _ _ _] -> [_ _ _ _ _ _ w685 _ _ _ _ _ _ _ _]
          seq-local: [_ _ _ _ _ _ w693 _ _ _ _ _ _ _ _] -> [_ _ _ _ _ _ _ _ w704 _ _ _ _ _ _]
          seq-local: [_ _ _ _ _ _ w692 _ _ _ _ _ _ _ _] -> [_ _ _ _ _ _ _ _ w703 _ _ _ _ _ _]
          seq-local: [_ _ _ _ _ _ _ _ w698 _ _ _ _ _ _] -> [_ _ _ _ _ _ _ _ _ _ w710 _ _ _ _]
          seq-local: [_ _ _ _ _ _ _ _ w697 _ _ _ _ _ _] -> [_ _ _ _ _ _ _ _ _ _ _ _ _ _ _]
          seq-local: [_ _ _ _ _ _ _ _ _ _ w706 _ _ _ _] -> [_ _ _ _ _ _ _ _ _ _ _ _ w720 _ _]
          seq-local: [_ _ _ _ _ _ _ _ _ _ w707 _ _ _ _] -> [_ _ _ _ _ _ _ _ _ _ _ _ w719 _ _]
          seq-local: [_ _ _ _ _ _ _ _ _ _ _ _ w718 _ _] -> [_ _ _ _ _ _ _ _ _ _ _ _ _ _ w733]
          seq-local: [_ _ _ _ _ _ _ _ _ _ _ _ w717 _ _] -> [_ _ _ _ _ _ _ _ _ _ _ _ _ _ w732]
          tunnel: w642 -> [w661 _ _ _ _ _ _ _ _ _ _ _ _ _ _]
          tunnel: w641 -> [w654 _ _ _ _ _ _ _ _ _ _ _ _ _ _]
          tunnel: w638 -> [w653 _ w667 _ w674 _ w690 _ w701 _ w711 _ w721 _ w728]
          tunnel: [_ _ _ _ _ _ _ _ _ _ _ _ _ _ w731] -> w640
          tunnel: [_ _ _ _ _ _ _ _ _ _ _ _ _ _ w730] -> w639
          tunnel: w637 -> [_ _ _ _ _ _ _ _ w695 _ _ _ _ _ _]
          frame #0 {
            w658 = " PULSe"  # Function Command
            n361 = Concatenate Strings(w653, ":FUNC" ("string (\"\")")) -> (w659:string)
            n362 = Pick Line(string ("")=w659, multi-line string=w658, line index="输出信号波形 2") -> (output string=w657:string)
            n363 = VISA Write(VISA resource name=w661, write buffer=w657, error in (no error)=w654) -> (VISA resource name out=w656:refnum<visa-resource-name>, error out=w655:errorcluster)  [unwired: 1 out]
          }
          frame #1 {
            n364 = Wait (ms)(milliseconds to wait=u32 150) -> ()  [unwired: 1 out]
          }
          frame #2 {
            n365 = Number To Fractional String(use system decimal point (T)=TRUE ("使用系统小数点(T)"), number="低电平/V 2") -> (F-format string=w665:string)  [unwired: 2 in]
            n366 = Concatenate Strings ("连接字符串")(w667, ":VOLTage:LOW ", w665) -> (w664:string)
            n367 = VISA Write(VISA resource name=w671, write buffer=w664, error in (no error)=w670) -> (VISA resource name out=w669:refnum<visa-resource-name>, error out=w668:errorcluster)  [unwired: 1 out]
          }
          frame #3 {
            n368 = Wait (ms)(milliseconds to wait=u32 150) -> ()  [unwired: 1 out]
          }
          frame #4 {
            # "1 频率"
            n369 = Concatenate Strings(w674, ":FREQ ") -> (w681:string)
            n370 = Format Into String ("格式化写入字符串")(initial string=w681, "频率/Hz 2") -> (resulting string=w682:string)  [unwired: 2 in, 1 out]
            n371 = VISA Write(VISA resource name=w680, write buffer=w682, error in (no error)=w679) -> (VISA resource name out=w678:refnum<visa-resource-name>, error out=w675:errorcluster)  [unwired: 1 out]
          }
          frame #5 {
            n372 = Wait (ms)(milliseconds to wait=u32 150) -> ()  [unwired: 1 out]
          }
          frame #6 {
            n373 = Number To Fractional String(use system decimal point (T)=TRUE ("使用系统小数点(T)"), number="高电平/V 2") -> (F-format string=w687:string)  [unwired: 2 in]
            n374 = Concatenate Strings(w690, ":VOLTage:HIGH ", w687) -> (w689:string)
            n375 = VISA Write(VISA resource name=w686, write buffer=w689, error in (no error)=w685) -> (VISA resource name out=w693:refnum<visa-resource-name>, error out=w692:errorcluster)  [unwired: 1 out]
          }
          frame #7 {
            n376 = Wait (ms)(milliseconds to wait=u32 150) -> ()  [unwired: 1 out]
          }
          frame #8 {
            n377 = Pick Line(multi-line string=":OUTP1:IMPedance \n:OUTP2:IMPedance " ("write buffer"), line index=w695) -> (output string=w699:string)  [unwired: 1 in]
            n378 = Concatenate Strings ("连接字符串")(w701, w699, "INFINITY") -> (w702:string)
            n379 = VISA Write(VISA resource name=w704, write buffer=w702, error in (no error)=w703) -> (VISA resource name out=w698:refnum<visa-resource-name>, error out=w697:errorcluster)  [unwired: 1 out]
          }
          frame #9 {
            n380 = Wait (ms)(milliseconds to wait=u32 150) -> ()  [unwired: 1 out]
          }
          frame #10 {
            n381 = Number To Fractional String(use system decimal point (T)=TRUE ("使用系统小数点(T)"), number="占空比/% 2") -> (F-format string=w713:string)  [unwired: 2 in]
            n382 = Concatenate Strings(w711, ":PULSe:DCYCle ", w713) -> (w708:string)
            n383 = VISA Write(VISA resource name=w710, write buffer=w708, error in (no error)=w709) -> (VISA resource name out=w706:refnum<visa-resource-name>, error out=w707:errorcluster)  [unwired: 1 out]
          }
          frame #11 {
            n384 = Wait (ms)(milliseconds to wait=u32 150) -> ()  [unwired: 1 out]
          }
          frame #12 {
            n385 = Number To Fractional String(use system decimal point (T)=TRUE ("使用系统小数点(T)"), number="延时/s 2") -> (F-format string=w724:string)  [unwired: 2 in]
            n386 = Concatenate Strings(w721, ":PULSe:DELay ", w724) -> (w722:string)
            n387 = VISA Write(VISA resource name=w720, write buffer=w722, error in (no error)=w719) -> (VISA resource name out=w718:refnum<visa-resource-name>, error out=w717:errorcluster)  [unwired: 1 out]
          }
          frame #13 {
            n388 = Wait (ms)(milliseconds to wait=u32 150) -> ()  [unwired: 1 out]
          }
          frame #14 {
            w736 = ":LEADing\n:TRAiling "  # Channel
            w740 = ":PULSe:TRANsition"  # VOLTage:Offset
            n389 = Pick Line(multi-line string=w736, line index="上升下降沿 2") -> (output string=w734:string)  [unwired: 1 in]
            n390 = Number To Fractional String(use system decimal point (T)=TRUE ("使用系统小数点(T)"), number="上升下降沿/s 2") -> (F-format string=w735:string)  [unwired: 2 in]
            n391 = Concatenate Strings(w728, w740, w734, w735) -> (w737:string)
            n392 = VISA Write(VISA resource name=w733, write buffer=w737, error in (no error)=w732) -> (VISA resource name out=w731:refnum<visa-resource-name>, error out=w730:errorcluster)  [unwired: 1 out]
          }
        }
        n393 = VISA Close(VISA resource name=w640, error in (no error)=w639) -> (error out=→"configure error out":errorcluster)
      }
    }
    n394 = event shown="[1] \"照明光\": 值改变" {
      selector: _ -> [_ _]
      dyn-events: _ -> [_ _]
      timeout: 0 -> [_ _]
      tunnel: "照明光" -> [_ w61]
      event Timeout {
        n395 = event-data() -> ()  [unwired: 1 in, 3 out]
      }
      event "照明光": Value Change {
        n396 = event-data() -> ()  [unwired: 1 in, 6 out]
        n397 = local read "stop bits (10: 1 bit)"() -> (w74:u16)
        n398 = local read "parity (0:none)"() -> (w73:enum16{"None", "Odd", "Even", "Mark", "Space"})
        n399 = local read "照明光VISA"() -> (w70:refnum<visa-resource-name>)
        n400 = local read "baud rate"() -> (w71:u32)
        n401 = local read "data bits (8)"() -> (w72:u16)
        n402 = call-poly "VISA Configure Serial Port"("VISA resource name"=w70, "baud rate (9600)"=w71, "data bits (8)"=w72, "parity (0:none)"=w73, "stop bits (10: 1 bit)"=w74) -> ("VISA resource name out"=w67:refnum<visa-resource-name>, "error out"=w66:errorcluster)  [unwired: 9 in]
        n403 = call <vilib>:"Simple Error Handler.vi"("error in (no error)"=w66) -> ()  [unwired: 4 in, 5 out]
        n404 = VISA Open(access mode=0, error in (no error)=w66, VISA resource name=w67) -> (VISA resource name=w69:refnum<visa-resource-name>, error out=w68:errorcluster)  [unwired: 2 in]
        n405 = stacked-sequence {
          tunnel: w69 -> [w79]
          tunnel: w68 -> [w78]
          tunnel: [w77] -> w64
          tunnel: [w76] -> w65
          tunnel: w61 -> [w75]
          frame #0 {
            n406 = case shown="假" w75 {
              tunnel: w79 -> [w85 w95]
              tunnel: [w83 w94] -> w77
              tunnel: w78 -> [w84 w93]
              tunnel: [w82 w92] -> w76
              frame False {
                n407 = Concatenate Strings(" \u0001\u0001¢", "\r") -> (w86:string)
                n408 = VISA Write(VISA resource name=w85, write buffer=w86, error in (no error)=w84) -> (VISA resource name out=w83:refnum<visa-resource-name>, error out=w82:errorcluster)  [unwired: 1 out]
                n409 = Wait (ms)(milliseconds to wait=50) -> ()  [unwired: 1 out]
              }
              frame True {
                w88 = " \u0001\u0000¡"  # Channel
                n410 = Wait (ms)(milliseconds to wait=50) -> ()  [unwired: 1 out]
                n411 = Concatenate Strings(w88, "\r") -> (w89:string)
                n412 = VISA Write(VISA resource name=w95, write buffer=w89, error in (no error)=w93) -> (VISA resource name out=w94:refnum<visa-resource-name>, error out=w92:errorcluster)  [unwired: 1 out]
              }
            }
          }
        }
        n413 = VISA Close(VISA resource name=w64, error in (no error)=w65) -> (error out=w63:errorcluster)
        n414 = call <vilib>:"Simple Error Handler.vi"("error in (no error)"=w63) -> ()  [unwired: 4 in, 5 out]
      }
    }
  }
  n415 = flat-sequence {
    frame #0 {
      "Backlight" <- i32[][] [] ("Backlight")
    }
    frame #1 {
      w831 = FALSE
      # "删除背景光控件\n初始值设定"
      n416 = local write "cut backlight"(w831) -> ()
      "backlight" <- w831
    }
  }
  n417 = stacked-sequence {
    seq-local: [_ _ _ w852 _ _ _ _] -> [_ _ _ _ w870 w890 w893 w1105]
    seq-local: [_ _ _ w851 _ _ _ _] -> [_ _ _ _ w871 w891 w892 w1106]
    frame #0 {
      # "initialize all variables"
      n418 = property on="initialize" class="Bool"("Désactivé"=u8 0) -> ()  [unwired: 2 in, 2 out]
      n419 = property on="Acquire" class="Bool"("Visible"=FALSE) -> ()  [unwired: 2 in, 2 out]
      n420 = property on="Setup" class="Bool"("Visible"=FALSE) -> ()  [unwired: 2 in, 2 out]
      n421 = local write "indicator"("" ("indicator")) -> ()
      n422 = local write "initialized ?"(FALSE ("initialized ?")) -> ()
      n423 = local write "Continuous"(FALSE ("Continuous")) -> ()
      n424 = local write "Close"(FALSE ("Close")) -> ()
      n425 = property on="Device Name" class="Ring (严格)"("Désactivé"=u8 0) -> ()  [unwired: 2 in, 2 out]
      n426 = property on="Continuous" class="Bool (严格)"("Visible"=FALSE) -> ()  [unwired: 2 in, 2 out]
      n427 = local write "Commande tab"(T1."Settings" ("Commande tab")) -> ()
    }
    frame #1 {
      # "Read Uniq ID"
      n428 = stacked-sequence {
        frame #0 {
          n429 = call "read detector uniq-id.vi"() -> ("nbr of components"=w844:i32, "UniqueID"=w843:string[], "Name"=w842:string[])  [unwired: 4 out]
          n430 = for {
            N: w844 -> [_]
            tunnel: w843 -> [w846]
            tunnel: w842 -> [w845]
            n431 = property on="Device Name" class="Ring (严格)"("Chaînes []"=w845) -> ()  [unwired: 2 in, 2 out]
            n432 = property on="Uniques ID" class="Ring (严格)"("Chaînes []"=w846) -> ()  [unwired: 2 in, 2 out]
          }
        }
      }
    }
    frame #2 {
      n433 = while {
        stop <- "initialize" stop-if-true
        n434 = local read "Device Name"() -> (w849:u16)
        n435 = local write "Uniques ID"(w849) -> ()
        n436 = local read "Close"() -> (w847:bool)
        n437 = Stop(stop? (T)=w847) -> ()
        n438 = Wait Until Next ms Multiple(millisecond multiple=u32 100 ("n millisecondes")) -> ()  [unwired: 1 out]
      }
    }
    frame #3 {
      n439 = stacked-sequence {
        tunnel: [_ w859 _ _] -> w852
        tunnel: [_ w858 _ _] -> w851
        frame #0 {
          n440 = local write "indicator"("Initializing ..." ("indicator")) -> ()
        }
        frame #1 {
          n441 = local read "Uniques ID"() -> (w856:u16)
          n442 = property on="Uniques ID" class="Ring (严格)"() -> ("Chaînes []"=w857:string[])  [unwired: 2 in, 2 out]
          n443 = Index Array(array=w857, index=w856) -> (element=w855:string)
          n444 = call "Initialize CCD.vi"("Unique id:"=w855) -> ("activeYPixels"=→"Y Pixels:":i32, "JYCCDLib.IJYCCDReqd"=w858:refnum<k7>, "activeXPixels"=→"X Pixels:":i32, "sortie d'erreur"=w859:errorcluster, "FirmwareVersion"=→"Firmware\nVersion":string)  [unwired: 3 out]
        }
        frame #2 {
          n445 = property on="initialize" class="Bool"("Désactivé"=u8 2) -> ()  [unwired: 2 in, 2 out]
          n446 = property on="Device Name" class="Ring (严格)"("Désactivé"=u8 2) -> ()  [unwired: 2 in, 2 out]
          n447 = local write "Continuous"(FALSE ("Continuous")) -> ()
          n448 = property on="Setup" class="Bool"("Visible"=TRUE) -> ()  [unwired: 2 in, 2 out]
        }
        frame #3 {
          n449 = local write "initialized ?"(TRUE ("initialized ?")) -> ()
          n450 = local write "indicator"("Initialized !" ("indicator")) -> ()
        }
      }
    }
    frame #4 {
      # "Actually not working"
      # "Read ADC and GAIN"
      n451 = case shown="真" "Constante de condition\n(Voir l'aide contextuelle)" {
        tunnel: w871 -> [_ w881]
        tunnel: w870 -> [_ w880]
        frame False {
        }
        frame True {
          # "Read Input supported trigger"
          n452 = call "Trigger - Get Supported Input.vi"("JYCCDLib.IJYCCDReqd"=w881, "Error Input"=w880) -> ("trigAddress"=w875:i32, "eventPtr"=w876:i32, "trigEventString"=w879:string, "trigSigType"=w878:i32, "trigSigTypeString"=w877:string)  [unwired: 4 out]
          n453 = local write "trigSigTypeString"(w877) -> ()
          n454 = local write "trigAddress"(w875) -> ()
          n455 = local write "Trigger Type :"(w876) -> ()
          n456 = local write "trigEventString"(w879) -> ()
          n457 = local write "Signal type :"(w878) -> ()
        }
      }
      n458 = call "Init ADC & Gain.vi"("JYCCDLib.IJYCCDReqd"=w871, "input error"=w870) -> ("ADC Number"=w869:i32[], "ADC description"=w874:string[], "Gain Number"=w872:i32[], "Gain description"=w873:string[])
      n459 = local write "Gain Number"(w872) -> ()
      n460 = local write "ADC Number"(w869) -> ()
      n461 = stacked-sequence {
        tunnel: w874 -> [w882 _]
        tunnel: w873 -> [_ w883]
        frame #0 {
          n462 = property on="ADC" class="Ring (严格)"("Chaînes []"=w882) -> ()  [unwired: 2 in, 2 out]
        }
        frame #1 {
          n463 = property on="GAIN" class="Ring (严格)"("Chaînes []"=w883) -> ()  [unwired: 2 in, 2 out]
        }
      }
    }
    frame #5 {
      # "IS multi Accumulation Supported ?"
      n464 = call "MultiAccu - Is Supported.vi"("Error In"=w890, "JYCCDLib.IJYCCDReqd"=w891) -> ("IsOperatingModeSupported"=w884:bool)  [unwired: 3 out]
      n465 = Select(t=0, s=w884, f=2) -> (s? t:f=w887:i32)
      n466 = Select(t=FALSE, s=w884, f=w884) -> (s? t:f=w886:bool)
      n467 = local write "Multi Accumulation mode:"(w886) -> ()
      n468 = property on="Multi Accumulation mode:" class="Bool (严格)"("Désactivé"=w887) -> ()  [unwired: 2 in, 2 out]
      n469 = property on="Multi Accumulation mode:" class="Bool (严格)"("Désactivé"=w887) -> ()  [unwired: 2 in, 2 out]
    }
    frame #6 {
      n470 = while {
        tunnel: w892 -> [w900]
        tunnel: w893 -> [w899]
        stop <- "Close" stop-if-true
        n471 = local read "Continuous"() -> (w901:bool)
        n472 = case shown="假" "Reformat" {
          frame False {
          }
          frame True {
            n473 = local read "Y Pixels:"() -> (w1083:i32)
            n474 = local read "X Pixels:"() -> (w1085:i32)
            n475 = call "Spectral Reformat CCD area.vi"("Y Pixels:"=w1083, "X Pixels:"=w1085, "numAreas"="Number of Areas :") -> ("areas :"=→"areas :":i32[][])  [unwired: 3 out]
          }
        }
        n476 = local read "Accumulations:"() -> (w896:u16)
        n477 = Or(x="Acquire", y=w901) -> (x .or. y?=w898:bool)
        n478 = case shown="真" w898 {
          tunnel: w900 -> [_ w913]
          tunnel: w899 -> [_ w912]
          tunnel: "Enable InputTriggers :" -> [_ w911]
          tunnel: "Multi Accumulation mode:" -> [_ w910]
          tunnel: w896 -> [_ w909]
          tunnel: "MultiAcqShutterMode" -> [_ w908]
          frame False {
          }
          frame True {
            n479 = stacked-sequence {
              seq-local: [_ _ w926 _ _ _] -> [_ _ _ w999 _ _]
              seq-local: [_ _ _ w972 _ _] -> [_ _ _ _ w1040 _]
              seq-local: [_ _ _ _ w1039 _] -> [_ _ _ _ _ w1069]
              tunnel: w913 -> [_ w915 w930 w998 _ _]
              tunnel: w912 -> [_ w916 w929 w997 _ _]
              tunnel: w911 -> [_ w917 _ _ _ _]
              tunnel: w910 -> [_ _ w928 _ _ _]
              tunnel: w909 -> [_ _ w927 _ _ _]
              tunnel: w908 -> [_ _ w925 _ _ _]
              frame #0 {
                n480 = local write "CCD Busy"(TRUE ("CCD Busy")) -> ()
              }
              frame #1 {
                n481 = case shown="真" w917 {
                  tunnel: w916 -> [w918 w924]
                  tunnel: w915 -> [w919 w923]
                  frame False {
                    n482 = call "Trigger - Disable.vi"("Error In"=w918, "JYCCDLib.IJYCCDReqd"=w919) -> ()  [unwired: 6 out]
                  }
                  frame True {
                    n483 = local read "Trigger Type :"() -> (w920:u16)
                    n484 = local read "Signal type :"() -> (w921:enum16{"TTL Rising Edge", "TTL Falling Edge"})
                    n485 = local read "trigAddress"() -> (w922:i32)
                    n486 = call "Trigger - Enable.vi"("Error In"=w924, "sigType"=w921, "event"=w920, "trigAddress"=w922, "JYCCDLib.IJYCCDReqd"=w923) -> ()  [unwired: 3 out]
                  }
                }
              }
              frame #2 {
                n487 = case shown="真" w928 {
                  selector: w928 -> [_ w959]
                  tunnel: w930 -> [w956 w962]
                  tunnel: w929 -> [w955 w961]
                  tunnel: w927 -> [_ w960]
                  tunnel: [u16 1 ("Accumulations:") w960] -> w926
                  tunnel: w925 -> [_ w958]
                  frame False {
                    n488 = call "MultiAccu - Disable.vi"("Error In"=w955, "JYCCDLib.IJYCCDReqd"=w956) -> ()  [unwired: 4 out]
                  }
                  frame True {
                    n489 = call "MultiAccu - Configure.vi"("JYCCDLib.IJYCCDReqd"=w962, "Cleans Before"="Number of Cleans", "Accumulations:"=w960, "MultiAcqHardwareMode"=w959, "MultiAcqShutterMode"=w958, "Error In"=w961) -> ()  [unwired: 1 in, 9 out]
                  }
                }
                n490 = flat-sequence {
                  frame #0 {
                    n491 = Current VI's Path() -> (path=w936:path)
                    n492 = Get Date/Time In Seconds() -> (seconds since 1Jan1904=w938:timestamp)
                    n493 = Strip Path(path=w936) -> (stripped path=w937:path)  [unwired: 1 out]
                    n494 = Path To String(path=w937) -> (string=w939:string)
                    n495 = Format Date/Time String(time format string (%c)="%m.%d" ("时间格式字符串(%c)"), seconds (now)=w938) -> (date/time string=w945:string)  [unwired: 1 in]
                    n496 = Concatenate Strings(w939, "\\Save\\" ("字符串"), w945) -> (w940:string)
                    n497 = String To Path(string=w940) -> (path=w941:path)
                    n498 = call <vilib>:"Check if File or Folder Exists.vi"("path"=w941) -> ("file or folder exists?"=w942:bool, "dup path"=w944:path)  [unwired: 8 in, 1 out]
                    n499 = case shown="真" w942 {
                      tunnel: [w952 w953] -> w943
                      tunnel: w944 -> [w951 w953]
                      tunnel: w945 -> [w950 _]
                      frame False {
                        n500 = Create Folder(prompt (Create Folder)=w950, path (use dialog)=w951) -> (created path=w952:path)  [unwired: 1 in, 2 out]
                      }
                      frame True {
                      }
                    }
                    n501 = Format Date/Time String(time format string (%c)="%y%m%d%H%M%S " ("时间格式字符串(%c)"), seconds (now)=w938) -> (date/time string=w948:string)  [unwired: 1 in]
                    n502 = Path To String(path=w943) -> (string=w946:string)
                    n503 = Concatenate Strings(w946, "\\" ("字符串")) -> (w947:string)
                    n504 = Concatenate Strings(w947, w948) -> (w935:string)
                    n505 = String To Path(string=w935) -> (path=→"最终存储路径 2":path)
                  }
                }
              }
              frame #3 {
                n506 = local read "cut backlight"() -> (w986:bool)
                n507 = local read "backlight"() -> (w985:bool)
                n508 = call "MultiAccu - Acquire spectral.vi"("error in"=w997, "Accumulations:"=w999, "ShutterOpen"="ShutterOpen", "JYCCDLib.IJYCCDReqd"=w998) -> ("Acq Time(ms)"=→"Acq Time(ms)":u32, "Array Out"=w996:i32[][][])  [unwired: 1 out]
                n509 = And(x=w986, y=w985) -> (x .and. y?=w987:bool)
                n510 = call "Array reset dimension.vi"("Area Number"="Area Number to Display", "Array In"=w996) -> ("Array Out"=w988:i32[][])
                n511 = case shown="真" w987 {
                  tunnel: [w1035 w1036] -> w989
                  tunnel: w988 -> [w1035 w1037]
                  frame False {
                  }
                  frame True {
                    n512 = local read "Backlight"() -> (w1038:i32[][])
                    n513 = Subtract(x=w1037, y=w1038) -> (x-y=w1036:i32[][])
                  }
                }
                n514 = local read "波长范围"() -> (w964:dbl[])
                n515 = local write "Data"(w988) -> ()
                n516 = Index Array(array=w989, index (row)=0 ("禁用的索引 (列)")) -> (element=w990:i32[])  [unwired: 1 in]
                n517 = Reverse 1D Array(array=w990) -> (reversed array=w973:i32[])
                n518 = call "转换至动态数据2"("Array"=w964) -> ("Dynamic Data Type"=w992:dynamicdata)  [unwired: 3 in]
                n519 = call "转换至动态数据"("Array"=w973) -> ("Dynamic Data Type"=w993:dynamicdata)  [unwired: 3 in]
                n520 = call <vilib>:"Median Filter.vi"("left rank"=6, "X"=w973) -> ("Filtered X"=w978:dbl[])  [unwired: 8 in, 1 out]
                n521 = call "Build XY Graph2"("Y Input"=w993, "X Input"=w992) -> ("XY Graph"=w991:cluster{"Y":dbl[], "Y":dbl[]}[])  [unwired: 8 in, 1 out]
                n522 = Subtract(x="拟合终点", y="拟合起点") -> (x-y=w967:i32)
                n523 = local write "Spectrum"(w991) -> ()
                n524 = local read "滤波阈值"() -> (w982:dbl)
                n525 = Array Subset(array=w964, index="拟合起点", length=w967) -> (w970:dbl[])
                n526 = local read "拟合参数"() -> (w963:dbl[])
                n527 = In Range and Coerce(upper limit=w982, x=w978, lower limit=-100.0) -> (In Range?=w981:bool[])  [unwired: 1 out]
                n528 = Not(x=w981) -> (.not. x?=w975:bool[])
                n529 = local read "滤波阈值"() -> (w977:dbl)
                n530 = local write "范围内？"(w981) -> ()
                n531 = local read "X Pixels:"() -> (w979:i32)
                n532 = Or Array Elements(Boolean array=w975) -> (logical OR=w980:bool)
                n533 = case shown="真" w980 {
                  tunnel: w979 -> [_ w1022]
                  tunnel: w978 -> [w1018 w1021]
                  tunnel: [w1018 w1020] -> w966
                  tunnel: w977 -> [_ w1019]
                  frame False {
                  }
                  frame True {
                    n534 = for {
                      N: w1022 -> [_]
                      tunnel: w1021 -> [w1026] mode=indexing
                      tunnel: [w1025] -> w1020 mode=indexing
                      shift-right: [w1025] -> _
                      shift-left: _ -> [w1024]
                      tunnel: w1019 -> [w1023]
                      n535 = Greater?(x=w1026, y=w1023) -> (0:w1028:bool)
                      n536 = Less?(x=w1026, y=-100.0) -> (x < y?=w1029:bool)
                      n537 = Or(x=w1028, y=w1029) -> (x .or. y?=w1027:bool)
                      n538 = case shown="真" w1027 {
                        tunnel: w1026 -> [w1031 _]
                        tunnel: [w1031 w1033] -> w1025
                        tunnel: w1024 -> [_ w1034]
                        frame False {
                        }
                        frame True {
                          n539 = call <vilib>:"Median Filter PtByPt.vi"("rank"=5, "x"=w1034) -> ("Filtered x"=w1033:dbl)  [unwired: 2 in, 1 out]
                        }
                      }
                    }
                  }
                }
                n540 = Array Subset(array=w966, index="拟合起点", length=w967) -> (w969:dbl[])
                n541 = Bundle("波长范围"=w964, "Filtered X"=w966) -> (w965:cluster{"波长范围 ":dbl[], "Filtered X":dbl[]})  [unwired: 1 in]
                n542 = case shown="真" "是否拟合" {
                  tunnel: w969 -> [w1002 w1008]
                  tunnel: w970 -> [_ w1007]
                  tunnel: [w1002 w1006] -> w984
                  tunnel: w965 -> [_ w1004]
                  frame False {
                  }
                  frame True {
                    n543 = call "转换至动态数据7"("Array"=w1008) -> ("Dynamic Data Type"=w1013:dynamicdata)  [unwired: 3 in]
                    n544 = call "转换至动态数据8"("Array"=w1007) -> ("Dynamic Data Type"=w1014:dynamicdata)  [unwired: 3 in]
                    n545 = call "曲线拟合2"("Locations"=w1014, "Signals"=w1013) -> ("best fit"=w1011:dynamicdata, "non-linear coefficients"=w1012:dynamicdata)  [unwired: 5 in, 3 out]
                    n546 = call "从动态数据转换3"("Dynamic Data Type"=w1012) -> ("Array"=w1015:dbl[])  [unwired: 3 in]
                    n547 = call "从动态数据转换4"("Dynamic Data Type"=w1011) -> ("Array"=w1006:dbl[])  [unwired: 3 in]
                    n548 = Index Array(array=w1015, index #1=0 ("索引"), index #2=1 ("索引")) -> (element #1=w1017:dbl, element #2=w1016:dbl)
                    n549 = local write "拟合参数"(w1015) -> ()
                    n550 = local write "xc"(w1017) -> ()
                    n551 = Bundle(w1007, "Array"=w1006) -> (w1005:cluster{dbl[], "Array":dbl[]})  [unwired: 1 in]
                    n552 = local write "w"(w1016) -> ()
                    n553 = Build Array(w1004, w1005) -> (→"best fit":cluster{"波长范围 ":dbl[], "Array":dbl[]}[])
                  }
                }
                n554 = Build Array(w970, w973, w984, w963) -> (w972:dbl[][])
              }
              frame #4 {
                n555 = case shown="假" "是否保存" {
                  tunnel: w1040 -> [_ w1046]
                  tunnel: ["0" w1045] -> w1039
                  frame False {
                  }
                  frame True {
                    n556 = Get Date/Time In Seconds() -> (seconds since 1Jan1904=w1060:timestamp)
                    n557 = Get Date/Time String(date format (0)=enum16{"short", "long", "abbreviated"}."abbreviated" ("日期格式(0)"), seconds (now)=w1060, want seconds? (F)=TRUE ("需要秒？(F)")) -> (date string=w1058:string, time string=w1059:string)
                    n558 = Search and Replace String(replace all?=TRUE ("替换全部？(F)"), input string=w1059, search string=":" ("搜索字符串"), replace string="-" ("替换字符串(\"\")")) -> (result string=w1057:string)  [unwired: 4 in, 3 out]
                    n559 = local read "最终存储路径 2"() -> (w1061:path)
                    n560 = Path To String(path=w1061) -> (string=w1063:string)
                    n561 = Concatenate Strings(w1063, w1058, w1057, "光谱" ("字符串"), ".xls" ("字符串")) -> (w1045:string)
                    n562 = String To Path(string=w1045) -> (path=w1062:path)
                    n563 = call-poly <vilib>:"Write Delimited Spreadsheet.vi"("file path (dialog if empty)"=w1062, "format (%.3f)"="%.16f", "2D data"=w1046, "append to file? (new file:F)"=TRUE ("append to file? (F)"), "transpose? (no:F)"=TRUE ("transpose? (F)")) -> ()  [unwired: 9 in, 2 out]
                  }
                }
                n564 = case shown="真" "Save Backlight" {
                  frame False {
                  }
                  frame True {
                    w1064 = TRUE ("删除背景光")
                    n565 = local read "Data"() -> (w1066:i32[][])
                    n566 = local write "Backlight"(w1066) -> ()
                    n567 = local write "cut backlight"(w1064) -> ()
                    n568 = local write "backlight"(w1064) -> ()
                    n569 = local write "Save Backlight"(FALSE ("Save Backlight")) -> ()
                  }
                }
                n570 = local write "CCD Busy"(FALSE ("CCD Busy")) -> ()
              }
              frame #5 {
                n571 = Open Python Session(python version="3.9" ("Python version")) -> (session out=w1073:refnum<k35>, error out=w1072:errorcluster)  [unwired: 2 in]
                n572 = node(w1073, path "D:/desktop/train/newpro_wan.py" ("module path"), "changexls2xlsx" ("function name"), w1072, w1069) -> (w1068:refnum<k35>, w1067:errorcluster)  [unwired: 3 in, 2 out]
                n573 = Close Python Session(session in=w1068, error in=w1067) -> ()  [unwired: 1 out]
              }
            }
          }
        }
        n574 = case shown="假" "Setup" {
          tunnel: w899 -> [_ w1088]
          tunnel: w900 -> [_ w1087]
          frame False {
          }
          frame True {
            n575 = stacked-sequence {
              tunnel: w1088 -> [_ w1102 _]
              tunnel: w1087 -> [_ w1090 _]
              frame #0 {
                n576 = local write "indicator"("Setting up the detector" ("indicator")) -> ()
              }
              frame #1 {
                w1100 = 1 items=["JYMCD_ACQ_FORMAT_IMAGE", "JYMCD_ACQ_FORMAT_SCAN"] ("Acquisition type")
                n577 = local read "Gain Number"() -> (w1095:i32[])
                n578 = local read "GAIN"() -> (w1091:u16)
                n579 = local read "ADC Number"() -> (w1096:i32[])
                n580 = local read "ADC"() -> (w1092:u16)
                n581 = Index Array(array=w1095, index=w1091) -> (element=w1093:i32)
                n582 = Index Array(array=w1096, index=w1092) -> (element=w1094:i32)
                n583 = local read "Number of Areas :"() -> (w1098:u16)
                n584 = local read "areas :"() -> (w1099:i32[][])
                n585 = call "Setup CCD.vi"("numAreas"=w1098, "areas :"=w1099, "JYCCDLib.IJYCCDReqd"=w1090, "entrée d'erreur (pas d'erreur)"=w1102, "Acquisition type"=w1100, "Gain"=w1093, "Select ADC"=w1094, "Integration time(ms)"="Integration time (ms) :") -> ("DataSize"=→"DataSize":i32)  [unwired: 1 out]
                "JYCCDLib.IJYCCDReqd" <- w1090
              }
              frame #2 {
                w1103 = TRUE ("Visible")
                n586 = property on="Continuous" class="Bool (严格)"("Visible"=w1103) -> ()  [unwired: 2 in, 2 out]
                n587 = property on="Acquire" class="Bool"("Visible"=w1103) -> ()  [unwired: 2 in, 2 out]
                n588 = local write "indicator"("Ready !" ("indicator")) -> ()
              }
            }
          }
        }
        n589 = case shown="假" "Temperature" {
          tunnel: w900 -> [_ w1077]
          tunnel: w899 -> [_ w1076]
          frame False {
            n590 = property on="temp graph" class="WFChart (严格)"("Visible"=FALSE) -> ()  [unwired: 2 in, 2 out]
          }
          frame True {
            n591 = stacked-sequence {
              tunnel: w1077 -> [_ w1082]
              tunnel: w1076 -> [_ w1081]
              frame #0 {
                n592 = property on="temp graph" class="WFChart (严格)"("Visible"=TRUE) -> ()  [unwired: 2 in, 2 out]
              }
              frame #1 {
                w1080 = u16 0 items=["° Celsius", "Kelvin", "° Farenheit"] ("units")
                n593 = call "read temperature.vi"("entrée d'erreur (pas d'erreur)"=w1081, "units"=w1080, "JYCCDLib.IJYCCDReqd"=w1082) -> ("Current Temperature"=w1079:dbl)
                n594 = local write "temp graph"(w1079) -> ()
              }
            }
          }
        }
        n595 = Wait Until Next ms Multiple(millisecond multiple=u32 50 ("n millisecondes")) -> ()  [unwired: 1 out]
      }
    }
    frame #7 {
      n596 = Close Reference(reference=w1106, error in (no error)=w1105) -> ()  [unwired: 1 out]
    }
  }
  n597 = stacked-sequence {
    seq-local: [_ _ w1116 _ _] -> [_ _ _ w1126 w1131]
    seq-local: [_ _ w1115 _ _] -> [_ _ _ w1125 _]
    seq-local: [_ _ _ w1124 _] -> [_ _ _ _ _]
    frame #0 {
      n598 = call "Get Monos From Config Browser.vi"() -> ("UniqueIDs"=w1111:string[], "Mono ID"=w1112:string[])  [unwired: 3 in, 1 out]
      n599 = Build Cluster Array(w1112, w1111) -> (w1109:cluster{"String":string, "String":string}[])
      n600 = property on="Mono ID" class="CmbBox"("Strings And Values []"=w1109) -> ()  [unwired: 2 in, 2 out]
      n601 = Index Array(array=w1109, index=0) -> (element=w1110:cluster{"String":string, "String":string})
      n602 = Unbundle(w1110) -> ("String"=w1107:string)  [unwired: 1 out]
      "Current UniqueID" <- w1107
      n603 = local write "Mono ID"(w1107) -> ()
    }
    frame #1 {
      n604 = while {
        stop <- "Connect" stop-if-true
        n605 = local read "Mono ID"() -> (w1113:string)
        n606 = local write "Current UniqueID"(w1113) -> ()
      }
    }
    frame #2 {
      n607 = local read "Mono ID"() -> (w1118:string)
      n608 = call "JYInitMono.vi"("Unique ID"=w1118, "Force Init"="Force\nInitialization") -> ("Refnum out"=w1116:refnum<k7>, "Initialized"=→"Initialized JY":bool, "error out"=w1115:errorcluster)  [unwired: 9 in, 2 out]
    }
    frame #3 {
      n609 = call "Show Current Grating.vi"("Refnum in"=w1126, "error in (no error)"=w1125) -> ("Gratings"=w1127:dbl[], "Grating Index"=w1121:i32, "Current Grating"=w1123:dbl, "Current Description"=w1120:string, "error out"=w1124:errorcluster)  [unwired: 5 in, 4 out]
      "Gratings" <- w1127
      n610 = local write "Current Grating"(w1123) -> ()
      n611 = local write "Current Description"(w1120) -> ()
      n612 = Number To Decimal String(number=w1127) -> (decimal integer string=w1129:string[])  [unwired: 1 in]
      n613 = Number To Decimal String(number=w1121) -> (decimal integer string=w1122:string)  [unwired: 1 in]
      n614 = property on="Target Grating" class="CmbBox"("Value"=w1122) -> ()  [unwired: 2 in, 2 out]
      n615 = Build Cluster Array(w1129, string[] ["1", "2", "3"]) -> (w1130:cluster{"Numeric":string, string}[])
      n616 = property on="Target Grating" class="CmbBox"("Strings And Values []"=w1130) -> ()  [unwired: 2 in, 2 out]
    }
    frame #4 {
      n617 = while {
        tunnel: w1131 -> [w1133]
        stop <- w1132 stop-if-true
        n618 = stacked-sequence {
          seq-local: [w1137 _ _ _ _] -> [_ w1144 w1155 _ w1163]
          seq-local: [w1136 _ _ _ _] -> [_ w1143 w1154 _ _]
          seq-local: [_ w1142 _ _ _] -> [_ _ _ _ _]
          seq-local: [_ w1141 _ _ _] -> [_ _ _ _ _]
          seq-local: [_ _ w1147 _ _] -> [_ _ _ _ _]
          seq-local: [_ _ w1146 _ _] -> [_ _ _ w1157 _]
          tunnel: w1133 -> [w1135 _ _ w1158 _]
          frame #0 {
            n619 = call "Show Current Grating.vi"("Refnum in"=w1135) -> ("Grating Index"=→"Grating Index":i32, "Current Grating"=→"Current Grating":dbl, "Current Description"=→"Current Description":string, "error out"=w1136:errorcluster, "JYMONOLib.IJYMonoReqd"=w1137:refnum<k7>)  [unwired: 6 in, 4 out]
          }
          frame #1 {
            n620 = call "JYGetCurrentWL.vi"("error in (no error)"=w1143, "JYMONOLib.IJYMonoReqd"=w1144) -> ("error out"=w1141:errorcluster, "Units"=→"Units":string, "Current WL"=→"Current WL":dbl, "JYMONOLib.IJYMonoReqd 2"=w1142:refnum<k7>)  [unwired: 6 in]
          }
          frame #2 {
            w1152 = u16 1 items=["Entrance", "Exit"] ("Mirror Number")
            w1153 = u16 0 items=["Entrance", "Exit"] ("Mirror Number")
            n621 = call "JYGetMirrorPos.vi"("error in (no error)"=w1154, "Mirror"=w1153, "Refnum In"=w1155) -> ("error out"=w1150:errorcluster, "Current Mirror Position"=→"Entrance Mirror\nPosition":i32, "Refnum Out"=w1151:refnum<k7>)  [unwired: 1 in]
            n622 = call "JYGetMirrorPos.vi"("error in (no error)"=w1150, "Mirror"=w1152, "Refnum In"=w1151) -> ("error out"=w1146:errorcluster, "Current Mirror Position"=→"Exit Mirror\nPosition":i32, "Refnum Out"=w1147:refnum<k7>)  [unwired: 1 in]
          }
          frame #3 {
            w1160 = u16 0 items=["Front Entrance", "Side Entrance", "Front Exit", "Side Exit", "First Intermediate", "Second Intermediate"] ("Slit")
            n623 = call "JYGetSlits.vi"("MonoRefNum IN"=w1158, "Slit"=w1160, "error in (no error)"=w1157) -> ("Units"=→"Units 2":string, "Slit Width"=→"Front Entrance":dbl, "error out"=→"error out":errorcluster)  [unwired: 13 in, 1 out]
          }
          frame #4 {
            n624 = case shown="假" "Move To\nTarget Positions" {
              tunnel: w1163 -> [_ w1164]
              frame False {
              }
              frame True {
                n625 = stacked-sequence {
                  seq-local: [w1166 _ _ _] -> [_ w1172 _ _]
                  seq-local: [_ w1170 _ _] -> [_ _ w1187 _]
                  seq-local: [_ _ w1174 _] -> [_ _ _ w1193]
                  seq-local: [_ _ _ w1190] -> [_ _ _ _]
                  tunnel: w1164 -> [w1168 w1171 w1185 w1194]
                  frame #0 {
                    n626 = property on="Target Grating" class="CmbBox"() -> ("Value"=w1165:string)  [unwired: 2 in, 2 out]
                    n627 = local read "error out"() -> (w1167:errorcluster)
                    n628 = Decimal String To Number(string=w1165) -> (number=w1169:i32)  [unwired: 2 in, 1 out]
                    n629 = call "JYTurret.vi"("error in (no error)"=w1167, "Grating Index"=w1169, "JYMONOLib.IJYMonoReqd"=w1168) -> ("error out"=w1166:errorcluster)  [unwired: 2 out]
                  }
                  frame #1 {
                    # "Move Grating to Target Position"
                    n630 = call "JYMoveToWavelength.vi"("error in (no error)"=w1172, "Target WL"="Target WL", "RefNum In"=w1171) -> ("error out"=w1170:errorcluster)  [unwired: 1 in, 2 out]
                  }
                  frame #2 {
                    w1180 = u16 1 items=["Entrance", "Exit"] ("Mirror Number")
                    w1179 = u16 0 items=["Entrance", "Exit"] ("Mirror Number")
                    w1186 = u16 1 items=["Entrance", "Exit", "Front", "Side"] ("Mirror Number")
                    w1189 = u16 0 items=["Entrance", "Exit", "Front", "Side"] ("Mirror Number")
                    # "Move Mirrors"
                    n631 = call "JYMirrorMove.vi"("error in (no error)"=w1187, "Mirror Position"="Entrance Mirror", "Mirror Number"=w1189, "RefNum In"=w1185) -> ("error out"=w1184:errorcluster)  [unwired: 6 in, 1 out]
                    n632 = call "JYMirrorMove.vi"("error in (no error)"=w1184, "Mirror Position"="Exit Mirror", "Mirror Number"=w1186, "RefNum In"=w1185) -> ("error out"=w1177:errorcluster, "MonoRefNum Out"=w1178:refnum<k7>)  [unwired: 6 in]
                    n633 = call "JYGetMirrorPos.vi"("error in (no error)"=w1177, "Mirror"=w1179, "Refnum In"=w1178) -> ("error out"=w1182:errorcluster, "Current Mirror Position"=w1176:i32, "Refnum Out"=w1181:refnum<k7>)  [unwired: 1 in]
                    n634 = local write "Entrance Mirror\nPosition"(w1176) -> ()
                    n635 = call "JYGetMirrorPos.vi"("error in (no error)"=w1182, "Mirror"=w1180, "Refnum In"=w1181) -> ("error out"=w1174:errorcluster, "Current Mirror Position"=w1175:i32)  [unwired: 1 in, 1 out]
                    n636 = local write "Exit Mirror\nPosition"(w1175) -> ()
                  }
                  frame #3 {
                    w1192 = u16 0 items=["Front Entrance", "Side Entrance", "Front Exit", "Side Exit", "First Intermediate", "Second Intermediate"] ("Slit")
                    # "Set New Slit Positions"
                    n637 = call "JYSlits.vi"("JYMONOLib.IJYMonoReqd"=w1194, "Slit"=w1192, "error in (no error)"=w1193, "Slit Width"="Target\nFront Entrance") -> ("error out"=w1190:errorcluster)  [unwired: 1 in, 1 out]
                  }
                }
              }
            }
          }
        }
        n638 = local read "Close"() -> (w1132:bool)
      }
    }
  }
  n639 = flat-sequence {
    frame #0 {
      n640 = call <vilib>:"Create Report.vi"("window state (normal)"=T3."no change", "report type"=Report_Type."Excel", "template (empty)"=path "D:/desktop/train/TEST1/Save/516中心波长.xlsx") -> ("report out"=w1201:refnum<class "NI_report.lvclass">, "error out"=w1200:errorcluster)  [unwired: 11 in]
      n641 = call-poly <vilib>:"Excel Get Data.vi"("report in"=w1201, "data type"=string[][] [], "error in (no error)"=w1200) -> ("report out"=w1196:refnum<class "NI_report.lvclass">, "data"=w1204:string[][], "error out"=w1195:errorcluster)  [unwired: 10 in]
      n642 = call-dynamic "Dispose Report.vi"("report in"=w1196, "error in (no error)"=w1195) -> ()  [unwired: 13 in, 1 out]
      n643 = Index Array(array=w1204, index (col)=0 ("禁用的索引 (列)")) -> (element=w1206:string[])  [unwired: 1 in]
      n644 = Fract/Exp String To Number(string=w1206) -> (number=→"波长范围":dbl[])  [unwired: 3 in, 1 out]
    }
  }
